vi "Autonomous Independent.vi"() -> ()   [LabVIEW 2023]
doc: "This VI is called when autonomous begins, and will automatically be terminated when autonomous ends. You can carry out timed or sensor driven robot movement independently without needing to return to the caller."
uses:
  <vilib>/Rock Robotics/WPI/ThirdParty/REV Robotics/REVLib/Typedef/Spark MAX Idle Mode.ctl
  <vilib>/Rock Robotics/WPI/SafetyOutput/WPI_SafetyOutputConfigMenu.ctl
  <vilib>/Rock Robotics/Network Tables/NT Read String.vi
  <vilib>/Rock Robotics/WPI/Utilities/WPI_GetSetVariantRefNum.vi
panel:
  out "Sensor Position 24":dbl
  out "Sensor Position 23":dbl
  out "Sensor Position 22":dbl
  out "Sensor Position 21":dbl
  out "Sensor Position 20":dbl
  out "Sensor Position 19":dbl
  out "Sensor Position 18":dbl
  out "Sensor Position 17":dbl
  out "Sensor Position 16":dbl
  out "Sensor Position 15":dbl
  out "Sensor Position 14":dbl
  out "Sensor Position 13":dbl
  out "Sensor Position 12":dbl
  out "Sensor Position 11":dbl
  out "Sensor Position 10":dbl
  out "Sensor Position 9":dbl
  out "Sensor Position 8":dbl
  out "Sensor Position 7":dbl
  out "?":dbl
  out "Sensor Position 6":dbl
  out "Sensor Position 5":dbl
  out "Sensor Position 4":dbl
  out "Sensor Position 3":dbl
  out "Sensor Position 2":dbl
  out "Sensor Position":dbl
  out "?":dbl
  # "Autonomous Independent.viBe sure to right-click and choose Data Operations>>Make Current Value default if you want to save the array values with the VI"
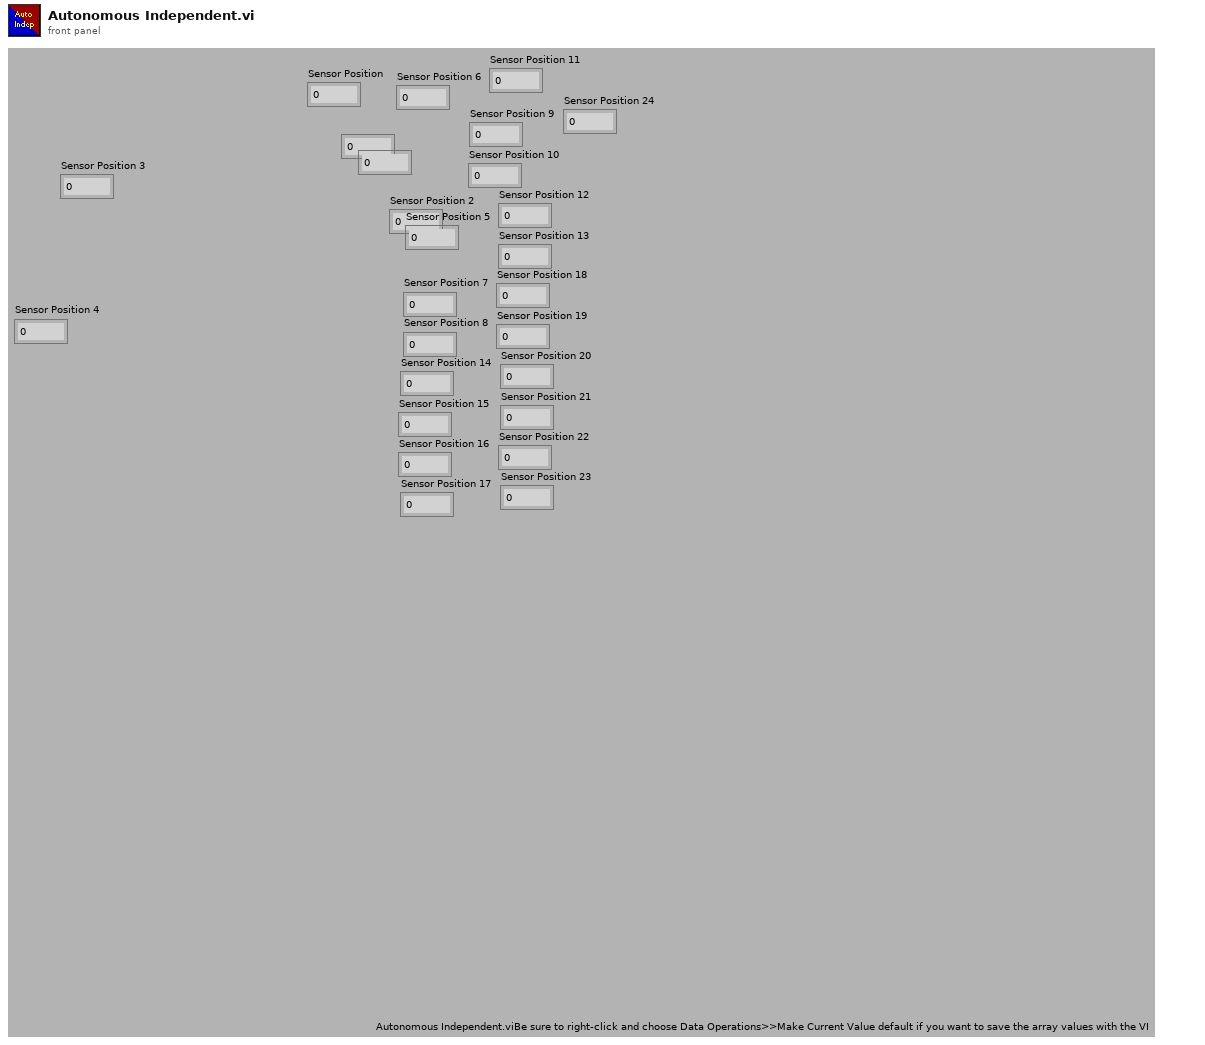
[diagram p1: front panel]
types:
  T1 = typedef "WPI_SafetyOutputConfigMenu.ctl" = enum16{"Enable", "Disable"}
  T2 = enum16{"ação 1", "ação 2", "ação 3", "ação 4", "ação 5", "ação 7", "ação 8"}
  T3 = typedef "Spark MAX Idle Mode.ctl" = enum16{"Coast", "Brake"}
  T4 = enum16{"ação 1", "ação 2", "ação 3", "ação 4", "ação 5"}
  T5 = typedef "WPI_RobotDriveDevRef.ctl" = cluster{"DevStatus":errorcluster, "Motors[]":T6[], "Square Inputs":bool, "Max Output":dbl}
  T6 = typedef "WPI_MotorControlDeviceRef.ctl" = cluster{"DeviceStatus":errorcluster, "Type":T7, "PWM":cluster{"PWM Channel":T8, "DeadBand":T9}, "CAN":cluster{"Device Number":u8, "SetOutput VI Ref":variant, "GetOutput VI Ref":variant, "Enable VI Ref":variant, "Disable VI Ref":variant, "Data":variant}, "Invert":bool, "DIO PWM":cluster{"PWM \"Enable\" Channel":T8, "DIOChannel":T10, "PWM Rate":dbl}}
  T7 = typedef "WPI_MotorControlType.ctl" = enum16{"PWM", "CAN", "DIO PWM"}
  T8 = typedef "FPGA_DIOPWMChannel.ctl" = enum8{"PWM 0", "PWM 1", "PWM 2", "PWM 3", "PWM 4", "PWM 5", "PWM 6", "PWM 7", "PWM 8", "PWM 9", "PWM MXP 0", "PWM MXP 1", "PWM MXP 2", "PWM MXP 3", "PWM MXP 4", "PWM MXP 5", "PWM MXP 6", "PWM MXP 7", "PWM MXP 8", "PWM MXP 9", "Invalid"}
  T9 = typedef "WPI_PWMDeadband.ctl" = cluster{"Name":string, "maxPositivePwm":i32, "minPositivePwm":i32, "centerPwm":i32, "maxNegativePwm":i32, "minNegativePwm":i32, "angularRange":u16}
  T10 = typedef "FPGA_DIOChannel.ctl" = enum8{"DIO 0", "DIO 1", "DIO 2", "DIO 3", "DIO 4", "DIO 5", "DIO 6", "DIO 7", "DIO 8", "DIO 9", "DIO MXP 0", "DIO MXP 1", "DIO MXP 2", "DIO MXP 3", "DIO MXP 4", "DIO MXP 5", "DIO MXP 6", "DIO MXP 7", "DIO MXP 8", "DIO MXP 9", "DIO MXP 10", "DIO MXP 11", "DIO MXP 12", "DIO MXP 13", "DIO MXP 14", "DIO MXP 15", "SPI Port CS1", "SPI Port CS2", "SPI Port CS3", "SPI Port MISO", "SPI Port MOSI", "Invalid"}
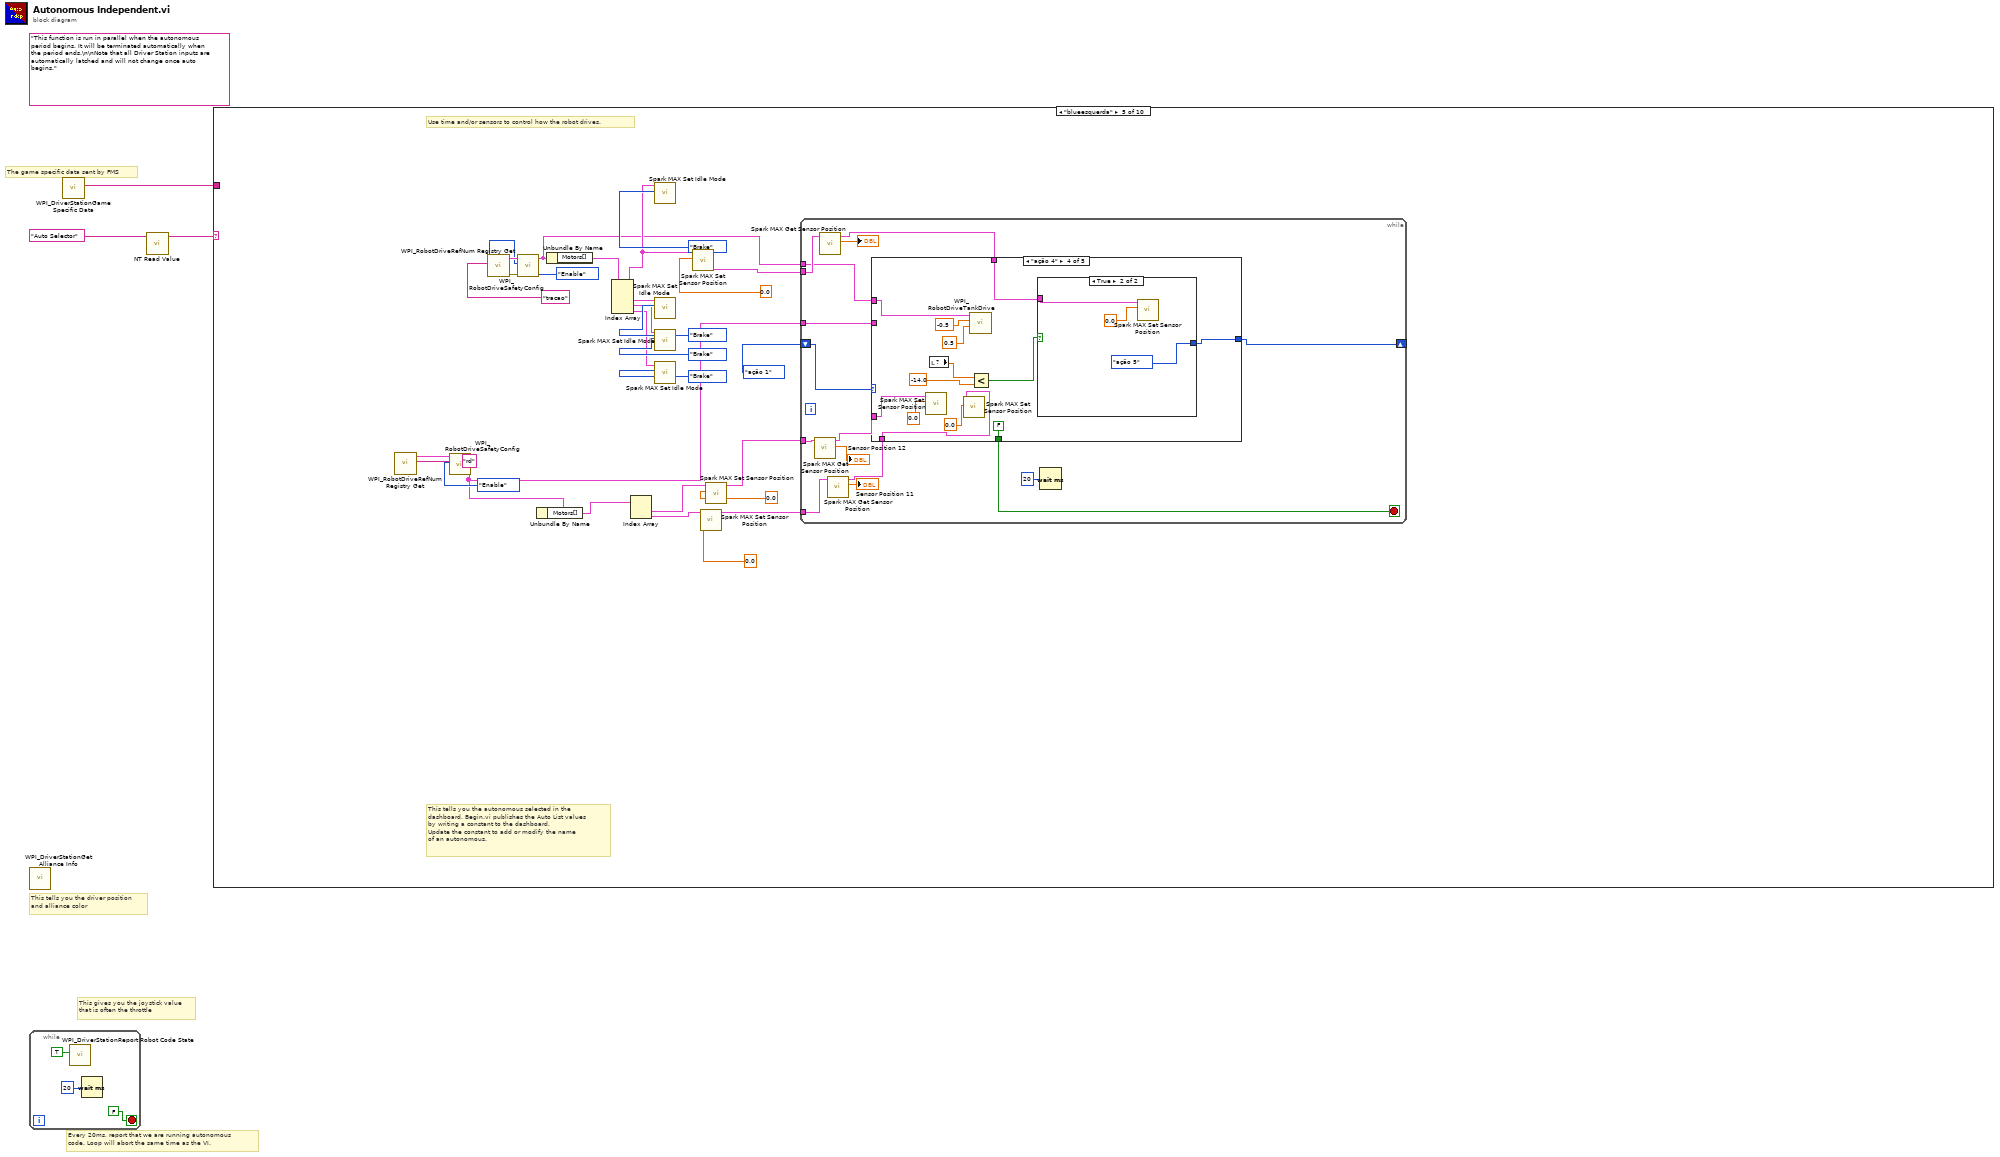
[diagram p0: block diagram]
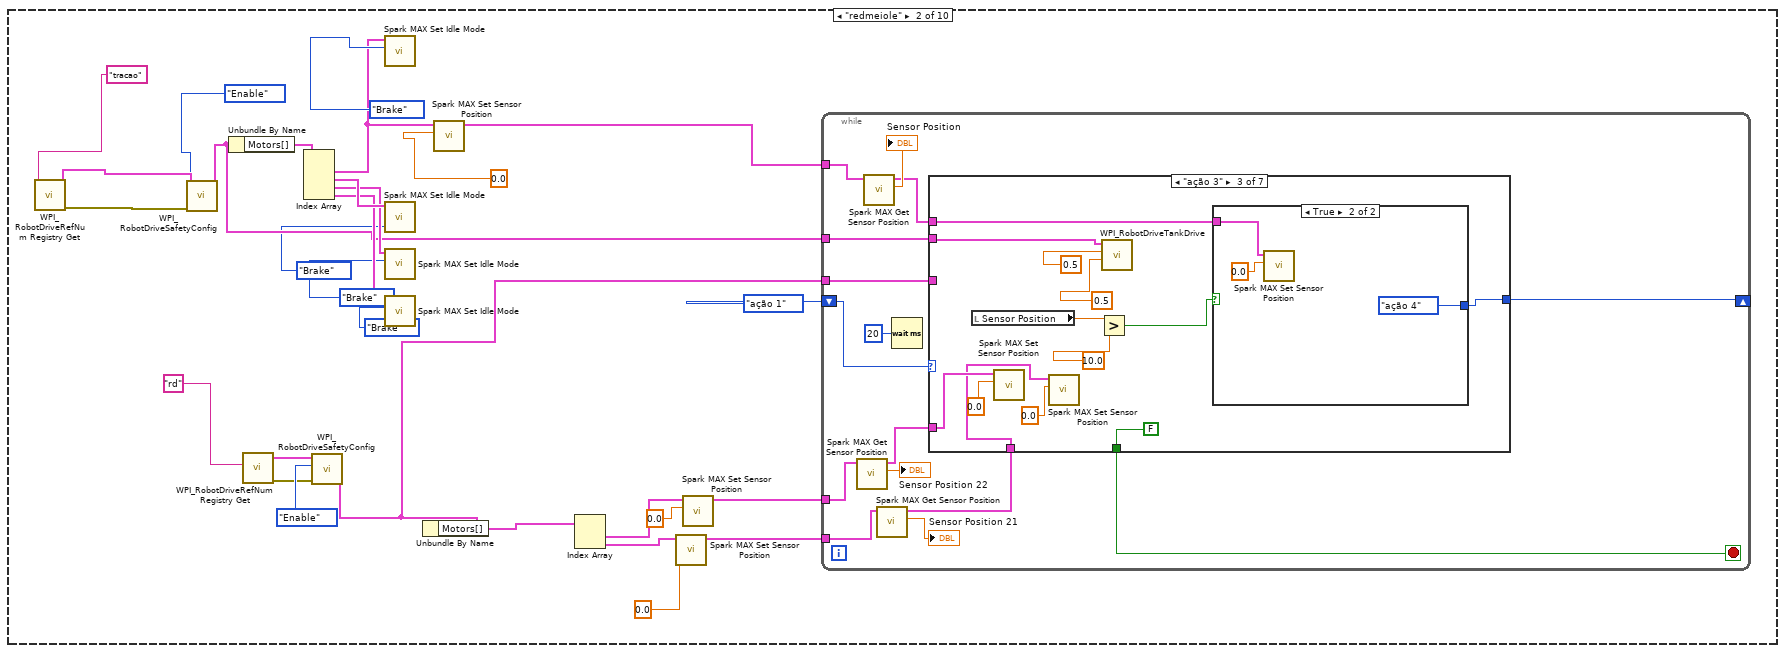
[diagram p3: hidden frame]
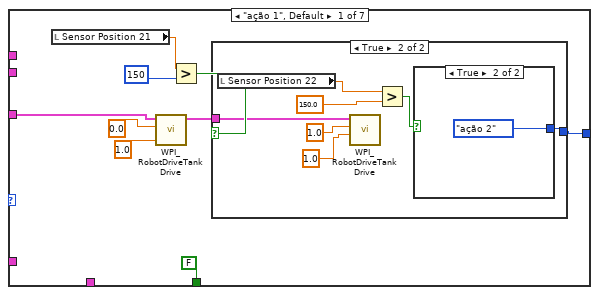
[diagram p4: hidden frame]
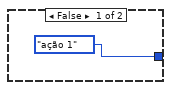
[diagram p5: hidden frame]
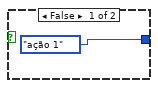
[diagram p6: hidden frame]
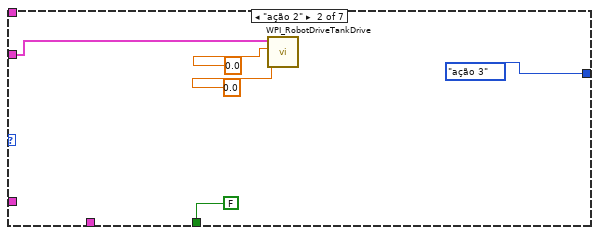
[diagram p7: hidden frame]
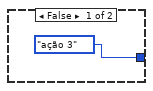
[diagram p8: hidden frame]
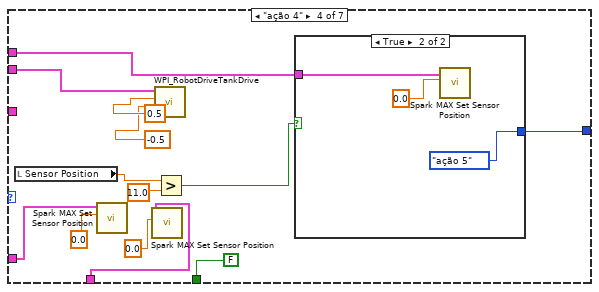
[diagram p9: hidden frame]
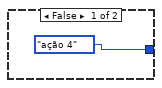
[diagram p10: hidden frame]
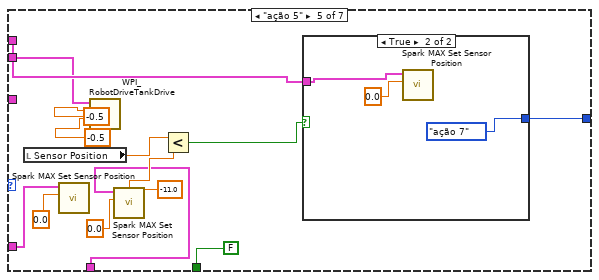
[diagram p11: hidden frame]
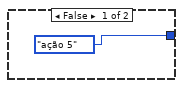
[diagram p12: hidden frame]
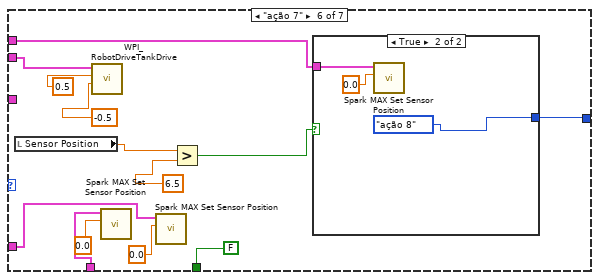
[diagram p13: hidden frame]
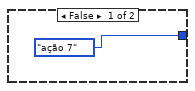
[diagram p14: hidden frame]
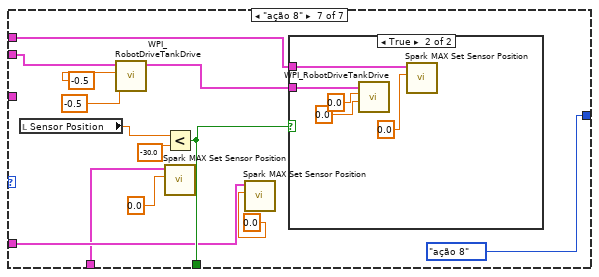
[diagram p15: hidden frame]
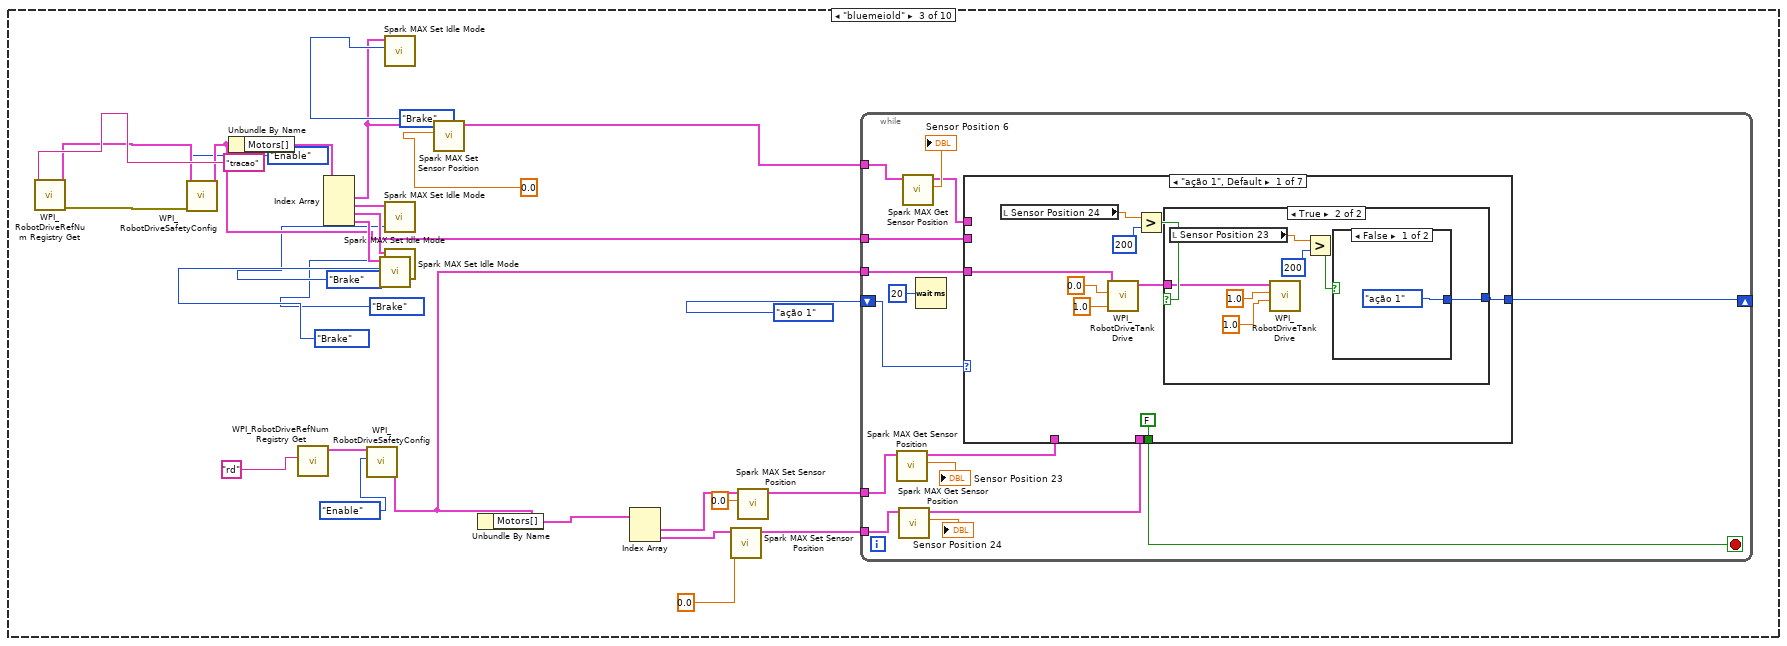
[diagram p17: hidden frame]
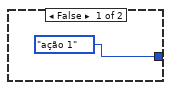
[diagram p18: hidden frame]
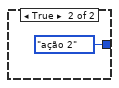
[diagram p19: hidden frame]
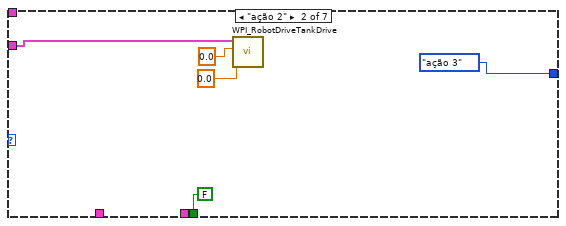
[diagram p20: hidden frame]
diagram:
  (unwired) "This function is run in parallel when the autonomous period begins. It will be terminated automatically when the period ends.\n\nNote that all Driver Station inputs are automatically latched and will not change once auto begins."
  # "The game specific data sent by FMS"
  # "This tells you the autonomous selected in the \ndashboard. Begin.vi publishes the Auto List values\nby writing a constant to the dashboard.\nUpdate the constant to add or modify the name\nof an autonomous."
  # "Every 20ms, report that we are running autonomous\ncode. Loop will abort the same time as the VI."
  # "This gives you the joystick value\nthat is often the throttle"
  # "Use time and/or sensors to control how the robot drives."
  # "This tells you the driver position\nand alliance color"
  n1 = call <vilib>:"WPI_DriverStationGet Alliance Info.vi"() -> ()  [unwired: 12 out]
  n2 = while {
    stop <- FALSE stop-if-true
    n3 = call <vilib>:"WPI_DriverStationReport Robot Code State.vi"("Autonomous"=TRUE) -> ()  [unwired: 10 in, 1 out]
    n4 = Wait (ms)(milliseconds to wait=u32 20) -> ()  [unwired: 1 out]
  }
  n5 = call <vilib>:"WPI_DriverStationGame Specific Data.vi"() -> ("Game Specific Data"=w1:string)  [unwired: 11 in]
  n6 = call-poly <vilib>:"NT Read Value.vi"("name"="Auto Selector" ("Name")) -> ("value"=w2:string)  [unwired: 8 in, 2 out]
  n7 = case shown="\"blueesquerda\"" w2 {
    tunnel: w1 -> [_ _ _ _ _ _ _ _ _ _]
    frame Default {
    }
    frame "redmeiole" {
      n8 = call <vilib>:"WPI_RobotDriveRefNum Registry Get.vi"("refnum name"="tracao") -> ("error out"=w34:errorcluster, "RobotDriveDevRef"=w33:T5)  [unwired: 9 in]
      n9 = call <vilib>:"WPI_RobotDriveSafetyConfig.vi"("error in (no error)"=w34, "mode"=WPI_SafetyOutputConfigMenu."Enable", "RobotDriveDevRef"=w33) -> ("RobotDriveDevRef"=w24:T5)  [unwired: 7 in, 1 out]
      n10 = Unbundle By Name(w24) -> ("Motors[]"=w32:T6[])
      n11 = call <vilib>:"WPI_RobotDriveRefNum Registry Get.vi"("refnum name"="rd") -> ("error out"=w7:errorcluster, "RobotDriveDevRef"=w13:T5)  [unwired: 9 in]
      n12 = Index Array(array=w32) -> (element #1=w25:T6, element #2=w29:T6, element #3=w28:T6, element #4=w27:T6)  [unwired: 4 in]
      n13 = call <vilib>:"WPI_RobotDriveSafetyConfig.vi"("error in (no error)"=w7, "mode"=WPI_SafetyOutputConfigMenu."Enable", "RobotDriveDevRef"=w13) -> ("RobotDriveDevRef"=w8:T5)  [unwired: 7 in, 1 out]
      n14 = call <vilib>:"Spark MAX Set Idle Mode.vi"("Idle Mode"=Spark_MAX_Idle_Mode."Brake", "MotorControlDeviceRef in"=w25) -> ()  [unwired: 8 in, 2 out]
      n15 = call <vilib>:"Spark MAX Set Idle Mode.vi"("Idle Mode"=Spark_MAX_Idle_Mode."Brake", "MotorControlDeviceRef in"=w29) -> ()  [unwired: 8 in, 2 out]
      n16 = call <vilib>:"Spark MAX Set Idle Mode.vi"("Idle Mode"=Spark_MAX_Idle_Mode."Brake", "MotorControlDeviceRef in"=w28) -> ()  [unwired: 8 in, 2 out]
      n17 = call <vilib>:"Spark MAX Set Idle Mode.vi"("Idle Mode"=Spark_MAX_Idle_Mode."Brake", "MotorControlDeviceRef in"=w27) -> ()  [unwired: 8 in, 2 out]
      n18 = Unbundle By Name(w8) -> ("Motors[]"=w18:T6[])
      n19 = call <vilib>:"Spark MAX Set Sensor Position.vi"("Position"=0.0, "MotorControlDeviceRef"=w25) -> ("MotorControlDeviceRef"=w23:T6)  [unwired: 8 in, 1 out]
      n20 = Index Array(array=w18) -> (element #1=w15:T6, element #2=w16:T6)  [unwired: 2 in]
      n21 = call <vilib>:"Spark MAX Set Sensor Position.vi"("Position"=0.0, "MotorControlDeviceRef"=w16) -> ("MotorControlDeviceRef"=w9:T6)  [unwired: 8 in, 1 out]
      n22 = call <vilib>:"Spark MAX Set Sensor Position.vi"("Position"=0.0, "MotorControlDeviceRef"=w15) -> ("MotorControlDeviceRef"=w10:T6)  [unwired: 8 in, 1 out]
      n23 = while {
        shift-right: [w48] -> _
        shift-left: T2."ação 1" -> [w49]
        tunnel: w24 -> [w47]
        tunnel: w23 -> [w45]
        tunnel: w10 -> [w42]
        tunnel: w9 -> [w41]
        tunnel: w8 -> [w38]
        stop <- w43 stop-if-true
        n24 = call <vilib>:"Spark MAX Get Sensor Position.vi"("MotorControlDevRef in"=w42) -> ("Sensor Position"=→"Sensor Position 22":dbl, "MotorControlDevRef out"=w37:T6)  [unwired: 7 in, 2 out]
        n25 = call <vilib>:"Spark MAX Get Sensor Position.vi"("MotorControlDevRef in"=w45) -> ("Sensor Position"=→"Sensor Position":dbl, "MotorControlDevRef out"=w44:T6)  [unwired: 7 in, 2 out]
        n26 = call <vilib>:"Spark MAX Get Sensor Position.vi"("MotorControlDevRef in"=w41) -> ("Sensor Position"=→"Sensor Position 21":dbl, "MotorControlDevRef out"=w36:T6)  [unwired: 7 in, 2 out]
        n27 = Wait (ms)(milliseconds to wait=u32 20) -> ()  [unwired: 1 out]
        n28 = case shown="\"ação 3\"" w49 {
          tunnel: [w54 T2."ação 3" w80 w97 w114 w131 T2."ação 8"] -> w48
          tunnel: w47 -> [_ _ w87 w104 w118 w138 w155]
          tunnel: w44 -> [_ _ w81 w98 w121 w132 w143]
          tunnel: [FALSE FALSE FALSE FALSE FALSE FALSE w149] -> w43
          tunnel: w38 -> [w51 w70 _ _ _ _ _]
          tunnel: w37 -> [_ _ w76 w92 w110 w126 w147]
          tunnel: w36 -> [_ _ w75 w93 w109 w127 w144]
          frame "ação 1", Default {
            n29 = local read "Sensor Position 21"() -> (w52:dbl)
            n30 = call <vilib>:"WPI_RobotDriveTankDrive.vi"("Right axis value"=1.0, "Left axis value"=0.0, "RobotDriveDevRef"=w51) -> ("RobotDriveDevRef"=w57:T5)  [unwired: 6 in, 2 out]
            n31 = Greater?(x=w52, y=u32 150) -> (0:w55:bool)
            n32 = case shown="True" w55 {
              tunnel: w57 -> [_ w65]
              tunnel: [T2."ação 1" w62] -> w54
              frame False {
              }
              frame True {
                n33 = local read "Sensor Position 22"() -> (w64:dbl)
                n34 = call <vilib>:"WPI_RobotDriveTankDrive.vi"("Right axis value"=1.0 ("Left axis value"), "Left axis value"=1.0 ("Right axis value"), "RobotDriveDevRef"=w65) -> ()  [unwired: 6 in, 3 out]
                n35 = Greater?(x=w64, y=150.0) -> (0:w63:bool)
                n36 = case shown="True" w63 {
                  tunnel: [T2."ação 1" T2."ação 2"] -> w62
                  frame False {
                  }
                  frame True {
                  }
                }
              }
            }
          }
          frame "ação 2" {
            n37 = call <vilib>:"WPI_RobotDriveTankDrive.vi"("Right axis value"=0.0, "Left axis value"=0.0, "RobotDriveDevRef"=w70) -> ()  [unwired: 6 in, 3 out]
          }
          frame "ação 3" {
            n38 = local read "Sensor Position"() -> (w83:dbl)
            n39 = call <vilib>:"Spark MAX Set Sensor Position.vi"("Position"=0.0, "MotorControlDeviceRef"=w76) -> ()  [unwired: 8 in, 2 out]
            n40 = call <vilib>:"Spark MAX Set Sensor Position.vi"("Position"=0.0, "MotorControlDeviceRef"=w75) -> ()  [unwired: 8 in, 2 out]
            n41 = Greater?(x=w83, y=10.0) -> (0:w84:bool)
            n42 = call <vilib>:"WPI_RobotDriveTankDrive.vi"("Right axis value"=0.5 ("Left axis value"), "Left axis value"=0.5, "RobotDriveDevRef"=w87) -> ()  [unwired: 6 in, 3 out]
            n43 = case shown="True" w84 {
              tunnel: w81 -> [_ w91]
              tunnel: [T2."ação 3" T2."ação 4"] -> w80
              frame False {
              }
              frame True {
                n44 = call <vilib>:"Spark MAX Set Sensor Position.vi"("Position"=0.0, "MotorControlDeviceRef"=w91) -> ()  [unwired: 8 in, 2 out]
              }
            }
          }
          frame "ação 4" {
            n45 = local read "Sensor Position"() -> (w101:dbl)
            n46 = call <vilib>:"Spark MAX Set Sensor Position.vi"("Position"=0.0, "MotorControlDeviceRef"=w92) -> ()  [unwired: 8 in, 2 out]
            n47 = call <vilib>:"Spark MAX Set Sensor Position.vi"("Position"=0.0, "MotorControlDeviceRef"=w93) -> ()  [unwired: 8 in, 2 out]
            n48 = call <vilib>:"WPI_RobotDriveTankDrive.vi"("Right axis value"=-0.5 ("Left axis value"), "Left axis value"=0.5, "RobotDriveDevRef"=w104) -> ()  [unwired: 6 in, 3 out]
            n49 = Greater?(x=w101, y=11.0) -> (0:w99:bool)
            n50 = case shown="True" w99 {
              tunnel: w98 -> [_ w108]
              tunnel: [T2."ação 4" T2."ação 5"] -> w97
              frame False {
              }
              frame True {
                n51 = call <vilib>:"Spark MAX Set Sensor Position.vi"("Position"=0.0, "MotorControlDeviceRef"=w108) -> ()  [unwired: 8 in, 2 out]
              }
            }
          }
          frame "ação 5" {
            n52 = local read "Sensor Position"() -> (w117:dbl)
            n53 = call <vilib>:"Spark MAX Set Sensor Position.vi"("Position"=0.0, "MotorControlDeviceRef"=w110) -> ()  [unwired: 8 in, 2 out]
            n54 = call <vilib>:"WPI_RobotDriveTankDrive.vi"("Right axis value"=-0.5 ("Left axis value"), "Left axis value"=-0.5, "RobotDriveDevRef"=w118) -> ()  [unwired: 6 in, 3 out]
            n55 = call <vilib>:"Spark MAX Set Sensor Position.vi"("Position"=0.0, "MotorControlDeviceRef"=w109) -> ()  [unwired: 8 in, 2 out]
            n56 = Less?(x=w117, y=-11.0) -> (x < y?=w115:bool)
            n57 = case shown="True" w115 {
              tunnel: w121 -> [_ w124]
              tunnel: [T2."ação 5" T2."ação 7"] -> w114
              frame False {
              }
              frame True {
                n58 = call <vilib>:"Spark MAX Set Sensor Position.vi"("Position"=0.0, "MotorControlDeviceRef"=w124) -> ()  [unwired: 8 in, 2 out]
              }
            }
          }
          frame "ação 7" {
            n59 = local read "Sensor Position"() -> (w135:dbl)
            n60 = call <vilib>:"WPI_RobotDriveTankDrive.vi"("Right axis value"=-0.5 ("Left axis value"), "Left axis value"=0.5, "RobotDriveDevRef"=w138) -> ()  [unwired: 6 in, 3 out]
            n61 = call <vilib>:"Spark MAX Set Sensor Position.vi"("Position"=0.0, "MotorControlDeviceRef"=w127) -> ()  [unwired: 8 in, 2 out]
            n62 = call <vilib>:"Spark MAX Set Sensor Position.vi"("Position"=0.0, "MotorControlDeviceRef"=w126) -> ()  [unwired: 8 in, 2 out]
            n63 = Greater?(x=w135, y=6.5) -> (0:w133:bool)
            n64 = case shown="True" w133 {
              tunnel: w132 -> [_ w142]
              tunnel: [T2."ação 7" T2."ação 8"] -> w131
              frame False {
              }
              frame True {
                n65 = call <vilib>:"Spark MAX Set Sensor Position.vi"("Position"=0.0, "MotorControlDeviceRef"=w142) -> ()  [unwired: 8 in, 2 out]
              }
            }
          }
          frame "ação 8" {
            n66 = local read "Sensor Position"() -> (w152:dbl)
            n67 = call <vilib>:"WPI_RobotDriveTankDrive.vi"("Right axis value"=-0.5 ("Left axis value"), "Left axis value"=-0.5, "RobotDriveDevRef"=w155) -> ("RobotDriveDevRef"=w150:T5)  [unwired: 6 in, 2 out]
            n68 = Less?(x=w152, y=-30.0) -> (x < y?=w149:bool)
            n69 = call <vilib>:"Spark MAX Set Sensor Position.vi"("Position"=0.0, "MotorControlDeviceRef"=w144) -> ()  [unwired: 8 in, 2 out]
            n70 = call <vilib>:"Spark MAX Set Sensor Position.vi"("Position"=0.0, "MotorControlDeviceRef"=w147) -> ()  [unwired: 8 in, 2 out]
            n71 = case shown="True" w149 {
              tunnel: w150 -> [_ w160]
              tunnel: w143 -> [_ w157]
              frame False {
              }
              frame True {
                n72 = call <vilib>:"WPI_RobotDriveTankDrive.vi"("Right axis value"=0.0 ("Left axis value"), "Left axis value"=0.0, "RobotDriveDevRef"=w160) -> ()  [unwired: 6 in, 3 out]
                n73 = call <vilib>:"Spark MAX Set Sensor Position.vi"("Position"=0.0, "MotorControlDeviceRef"=w157) -> ()  [unwired: 8 in, 2 out]
              }
            }
          }
        }
      }
    }
    frame "bluemeiold" {
      n74 = call <vilib>:"WPI_RobotDriveRefNum Registry Get.vi"("refnum name"="tracao") -> ("error out"=w187:errorcluster, "RobotDriveDevRef"=w186:T5)  [unwired: 9 in]
      n75 = call <vilib>:"WPI_RobotDriveSafetyConfig.vi"("error in (no error)"=w187, "mode"=WPI_SafetyOutputConfigMenu."Enable", "RobotDriveDevRef"=w186) -> ("RobotDriveDevRef"=w177:T5)  [unwired: 7 in, 1 out]
      n76 = Unbundle By Name(w177) -> ("Motors[]"=w185:T6[])
      n77 = call <vilib>:"WPI_RobotDriveRefNum Registry Get.vi"("refnum name"="rd") -> ("RobotDriveDevRef"=w165:T5)  [unwired: 9 in, 1 out]
      n78 = Index Array(array=w185) -> (element #1=w178:T6, element #2=w182:T6, element #3=w181:T6, element #4=w180:T6)  [unwired: 4 in]
      n79 = call <vilib>:"WPI_RobotDriveSafetyConfig.vi"("mode"=WPI_SafetyOutputConfigMenu."Enable", "RobotDriveDevRef"=w165) -> ("RobotDriveDevRef"=w161:T5)  [unwired: 8 in, 1 out]
      n80 = call <vilib>:"Spark MAX Set Idle Mode.vi"("Idle Mode"=Spark_MAX_Idle_Mode."Brake", "MotorControlDeviceRef in"=w180) -> ()  [unwired: 8 in, 2 out]
      n81 = call <vilib>:"Spark MAX Set Idle Mode.vi"("Idle Mode"=Spark_MAX_Idle_Mode."Brake", "MotorControlDeviceRef in"=w178) -> ()  [unwired: 8 in, 2 out]
      n82 = call <vilib>:"Spark MAX Set Idle Mode.vi"("Idle Mode"=Spark_MAX_Idle_Mode."Brake", "MotorControlDeviceRef in"=w182) -> ()  [unwired: 8 in, 2 out]
      n83 = call <vilib>:"Spark MAX Set Idle Mode.vi"("Idle Mode"=Spark_MAX_Idle_Mode."Brake", "MotorControlDeviceRef in"=w181) -> ()  [unwired: 8 in, 2 out]
      n84 = call <vilib>:"Spark MAX Set Sensor Position.vi"("Position"=0.0, "MotorControlDeviceRef"=w178) -> ("MotorControlDeviceRef"=w176:T6)  [unwired: 8 in, 1 out]
      n85 = Unbundle By Name(w161) -> ("Motors[]"=w171:T6[])
      n86 = Index Array(array=w171) -> (element #1=w168:T6, element #2=w169:T6)  [unwired: 2 in]
      n87 = call <vilib>:"Spark MAX Set Sensor Position.vi"("Position"=0.0, "MotorControlDeviceRef"=w169) -> ("MotorControlDeviceRef"=w162:T6)  [unwired: 8 in, 1 out]
      n88 = call <vilib>:"Spark MAX Set Sensor Position.vi"("Position"=0.0, "MotorControlDeviceRef"=w168) -> ("MotorControlDeviceRef"=w163:T6)  [unwired: 8 in, 1 out]
      n89 = while {
        shift-right: [w201] -> _
        shift-left: T2."ação 1" -> [w202]
        tunnel: w177 -> [w200]
        tunnel: w176 -> [w198]
        tunnel: w163 -> [w195]
        tunnel: w162 -> [w194]
        tunnel: w161 -> [w191]
        stop <- w196 stop-if-true
        n90 = call <vilib>:"Spark MAX Get Sensor Position.vi"("MotorControlDevRef in"=w195) -> ("Sensor Position"=→"Sensor Position 23":dbl, "MotorControlDevRef out"=w190:T6)  [unwired: 7 in, 2 out]
        n91 = call <vilib>:"Spark MAX Get Sensor Position.vi"("MotorControlDevRef in"=w194) -> ("Sensor Position"=→"Sensor Position 24":dbl, "MotorControlDevRef out"=w189:T6)  [unwired: 7 in, 2 out]
        n92 = call <vilib>:"Spark MAX Get Sensor Position.vi"("MotorControlDevRef in"=w198) -> ("Sensor Position"=→"Sensor Position 6":dbl, "MotorControlDevRef out"=w197:T6)  [unwired: 7 in, 2 out]
        n93 = Wait (ms)(milliseconds to wait=u32 20) -> ()  [unwired: 1 out]
        n94 = case shown="\"ação 1\", Default" w202 {
          tunnel: [w207 T2."ação 3" w233 w250 w267 w284 T2."ação 8"] -> w201
          tunnel: w200 -> [_ _ w240 w257 w271 w291 w308]
          tunnel: w197 -> [_ _ w234 w251 w274 w285 w296]
          tunnel: [FALSE FALSE FALSE FALSE FALSE FALSE w302] -> w196
          tunnel: w191 -> [w204 w223 _ _ _ _ _]
          tunnel: w190 -> [_ _ w229 w246 w265 w282 w298]
          tunnel: w189 -> [_ _ w228 w245 w264 w281 w297]
          frame "ação 1", Default {
            n95 = local read "Sensor Position 24"() -> (w205:dbl)
            n96 = call <vilib>:"WPI_RobotDriveTankDrive.vi"("Right axis value"=1.0, "Left axis value"=0.0, "RobotDriveDevRef"=w204) -> ("RobotDriveDevRef"=w210:T5)  [unwired: 6 in, 2 out]
            n97 = Greater?(x=w205, y=u32 200) -> (0:w208:bool)
            n98 = case shown="True" w208 {
              tunnel: w210 -> [_ w218]
              tunnel: [T2."ação 1" w214] -> w207
              frame False {
              }
              frame True {
                n99 = local read "Sensor Position 23"() -> (w217:dbl)
                n100 = call <vilib>:"WPI_RobotDriveTankDrive.vi"("Right axis value"=1.0 ("Left axis value"), "Left axis value"=1.0 ("Right axis value"), "RobotDriveDevRef"=w218) -> ()  [unwired: 6 in, 3 out]
                n101 = Greater?(x=w217, y=u32 200) -> (0:w215:bool)
                n102 = case shown="False" w215 {
                  tunnel: [T2."ação 1" T2."ação 2"] -> w214
                  frame False {
                  }
                  frame True {
                  }
                }
              }
            }
          }
          frame "ação 2" {
            n103 = call <vilib>:"WPI_RobotDriveTankDrive.vi"("Right axis value"=0.0, "Left axis value"=0.0, "RobotDriveDevRef"=w223) -> ()  [unwired: 6 in, 3 out]
          }
          frame "ação 3" {
            n104 = local read "Sensor Position 6"() -> (w236:dbl)
            n105 = call <vilib>:"Spark MAX Set Sensor Position.vi"("Position"=0.0, "MotorControlDeviceRef"=w229) -> ()  [unwired: 8 in, 2 out]
            n106 = Greater?(x=w236, y=10.0) -> (0:w237:bool)
            n107 = call <vilib>:"WPI_RobotDriveTankDrive.vi"("Right axis value"=0.5 ("Left axis value"), "Left axis value"=0.5, "RobotDriveDevRef"=w240) -> ()  [unwired: 6 in, 3 out]
            n108 = call <vilib>:"Spark MAX Set Sensor Position.vi"("Position"=0.0, "MotorControlDeviceRef"=w228) -> ()  [unwired: 8 in, 2 out]
            n109 = case shown="True" w237 {
              tunnel: w234 -> [_ w244]
              tunnel: [T2."ação 3" T2."ação 4"] -> w233
              frame False {
              }
              frame True {
                n110 = call <vilib>:"Spark MAX Set Sensor Position.vi"("Position"=0.0, "MotorControlDeviceRef"=w244) -> ()  [unwired: 8 in, 2 out]
              }
            }
          }
          frame "ação 4" {
            n111 = local read "Sensor Position 6"() -> (w254:dbl)
            n112 = call <vilib>:"WPI_RobotDriveTankDrive.vi"("Right axis value"=0.5 ("Left axis value"), "Left axis value"=-0.5, "RobotDriveDevRef"=w257) -> ()  [unwired: 6 in, 3 out]
            n113 = Less?(x=w254, y=-11.0) -> (x < y?=w252:bool)
            n114 = call <vilib>:"Spark MAX Set Sensor Position.vi"("Position"=0.0, "MotorControlDeviceRef"=w246) -> ()  [unwired: 8 in, 2 out]
            n115 = call <vilib>:"Spark MAX Set Sensor Position.vi"("Position"=0.0, "MotorControlDeviceRef"=w245) -> ()  [unwired: 8 in, 2 out]
            n116 = case shown="True" w252 {
              tunnel: w251 -> [_ w261]
              tunnel: [T2."ação 4" T2."ação 5"] -> w250
              frame False {
              }
              frame True {
                n117 = call <vilib>:"Spark MAX Set Sensor Position.vi"("Position"=0.0, "MotorControlDeviceRef"=w261) -> ()  [unwired: 8 in, 2 out]
              }
            }
          }
          frame "ação 5" {
            n118 = local read "Sensor Position 6"() -> (w270:dbl)
            n119 = call <vilib>:"WPI_RobotDriveTankDrive.vi"("Right axis value"=-0.5 ("Left axis value"), "Left axis value"=-0.5, "RobotDriveDevRef"=w271) -> ()  [unwired: 6 in, 3 out]
            n120 = Less?(x=w270, y=-11.0) -> (x < y?=w268:bool)
            n121 = call <vilib>:"Spark MAX Set Sensor Position.vi"("Position"=0.0, "MotorControlDeviceRef"=w265) -> ()  [unwired: 8 in, 2 out]
            n122 = call <vilib>:"Spark MAX Set Sensor Position.vi"("Position"=0.0, "MotorControlDeviceRef"=w264) -> ()  [unwired: 8 in, 2 out]
            n123 = case shown="True" w268 {
              tunnel: w274 -> [_ w277]
              tunnel: [T2."ação 5" T2."ação 7"] -> w267
              frame False {
              }
              frame True {
                n124 = call <vilib>:"Spark MAX Set Sensor Position.vi"("Position"=0.0, "MotorControlDeviceRef"=w277) -> ()  [unwired: 8 in, 2 out]
              }
            }
          }
          frame "ação 7" {
            n125 = local read "Sensor Position 6"() -> (w288:dbl)
            n126 = call <vilib>:"WPI_RobotDriveTankDrive.vi"("Right axis value"=0.5 ("Left axis value"), "Left axis value"=-0.5, "RobotDriveDevRef"=w291) -> ()  [unwired: 6 in, 3 out]
            n127 = Less?(x=w288, y=-6.5) -> (x < y?=w286:bool)
            n128 = call <vilib>:"Spark MAX Set Sensor Position.vi"("Position"=0.0, "MotorControlDeviceRef"=w282) -> ()  [unwired: 8 in, 2 out]
            n129 = call <vilib>:"Spark MAX Set Sensor Position.vi"("Position"=0.0, "MotorControlDeviceRef"=w281) -> ()  [unwired: 8 in, 2 out]
            n130 = case shown="True" w286 {
              tunnel: w285 -> [_ w295]
              tunnel: [T2."ação 7" T2."ação 8"] -> w284
              frame False {
              }
              frame True {
                n131 = call <vilib>:"Spark MAX Set Sensor Position.vi"("Position"=0.0, "MotorControlDeviceRef"=w295) -> ()  [unwired: 8 in, 2 out]
              }
            }
          }
          frame "ação 8" {
            n132 = local read "Sensor Position 6"() -> (w305:dbl)
            n133 = call <vilib>:"Spark MAX Set Sensor Position.vi"("Position"=0.0, "MotorControlDeviceRef"=w298) -> ()  [unwired: 8 in, 2 out]
            n134 = call <vilib>:"WPI_RobotDriveTankDrive.vi"("Right axis value"=-0.5 ("Left axis value"), "Left axis value"=-0.5, "RobotDriveDevRef"=w308) -> ("RobotDriveDevRef"=w303:T5)  [unwired: 6 in, 2 out]
            n135 = Less?(x=w305, y=-30.0) -> (x < y?=w302:bool)
            n136 = call <vilib>:"Spark MAX Set Sensor Position.vi"("Position"=0.0, "MotorControlDeviceRef"=w297) -> ()  [unwired: 8 in, 2 out]
            n137 = case shown="True" w302 {
              tunnel: w303 -> [_ w313]
              tunnel: w296 -> [_ w310]
              frame False {
              }
              frame True {
                n138 = call <vilib>:"WPI_RobotDriveTankDrive.vi"("Right axis value"=0.0 ("Left axis value"), "Left axis value"=0.0, "RobotDriveDevRef"=w313) -> ()  [unwired: 6 in, 3 out]
                n139 = call <vilib>:"Spark MAX Set Sensor Position.vi"("Position"=0.0, "MotorControlDeviceRef"=w310) -> ()  [unwired: 8 in, 2 out]
              }
            }
          }
        }
      }
    }
    frame "reddireita" {
      n140 = call <vilib>:"WPI_RobotDriveRefNum Registry Get.vi"("refnum name"="rd") -> ("RobotDriveDevRef"=w323:T5)  [unwired: 9 in, 1 out]
      n141 = call <vilib>:"WPI_RobotDriveSafetyConfig.vi"("mode"=WPI_SafetyOutputConfigMenu."Enable", "RobotDriveDevRef"=w323) -> ("RobotDriveDevRef"=w314:T5)  [unwired: 8 in, 1 out]
      n142 = call <vilib>:"WPI_RobotDriveRefNum Registry Get.vi"("refnum name"="tracao") -> ("error out"=w340:errorcluster, "RobotDriveDevRef"=w339:T5)  [unwired: 9 in]
      n143 = call <vilib>:"WPI_RobotDriveSafetyConfig.vi"("error in (no error)"=w340, "mode"=WPI_SafetyOutputConfigMenu."Enable", "RobotDriveDevRef"=w339) -> ("RobotDriveDevRef"=w325:T5)  [unwired: 7 in, 1 out]
      n144 = Unbundle By Name(w314) -> ("Motors[]"=w321:T6[])
      n145 = Unbundle By Name(w325) -> ("Motors[]"=w337:T6[])
      n146 = Index Array(array=w337) -> (element #1=w329:T6, element #2=w332:T6, element #3=w331:T6, element #4=w330:T6)  [unwired: 4 in]
      n147 = Index Array(array=w321) -> (element #1=w317:T6, element #2=w318:T6)  [unwired: 2 in]
      n148 = call <vilib>:"Spark MAX Set Idle Mode.vi"("Idle Mode"=Spark_MAX_Idle_Mode."Brake", "MotorControlDeviceRef in"=w329) -> ()  [unwired: 8 in, 2 out]
      n149 = call <vilib>:"Spark MAX Set Idle Mode.vi"("Idle Mode"=Spark_MAX_Idle_Mode."Brake", "MotorControlDeviceRef in"=w332) -> ()  [unwired: 8 in, 2 out]
      n150 = call <vilib>:"Spark MAX Set Idle Mode.vi"("Idle Mode"=Spark_MAX_Idle_Mode."Brake", "MotorControlDeviceRef in"=w331) -> ()  [unwired: 8 in, 2 out]
      n151 = call <vilib>:"Spark MAX Set Idle Mode.vi"("Idle Mode"=Spark_MAX_Idle_Mode."Brake", "MotorControlDeviceRef in"=w330) -> ()  [unwired: 8 in, 2 out]
      n152 = call <vilib>:"Spark MAX Set Sensor Position.vi"("Position"=0.0, "MotorControlDeviceRef"=w329) -> ("MotorControlDeviceRef"=w327:T6)  [unwired: 8 in, 1 out]
      n153 = call <vilib>:"Spark MAX Set Sensor Position.vi"("Position"=0.0, "MotorControlDeviceRef"=w318) -> ("MotorControlDeviceRef"=w319:T6)  [unwired: 8 in, 1 out]
      n154 = call <vilib>:"Spark MAX Set Sensor Position.vi"("Position"=0.0, "MotorControlDeviceRef"=w317) -> ("MotorControlDeviceRef"=w315:T6)  [unwired: 8 in, 1 out]
      n155 = while {
        shift-right: [w350] -> _
        shift-left: T4."ação 1" -> [w355]
        tunnel: w327 -> [w353]
        tunnel: w325 -> [w351]
        tunnel: w319 -> [w348]
        tunnel: w315 -> [w346]
        tunnel: w314 -> [w344]
        stop <- w354 stop-if-true
        n156 = call <vilib>:"Spark MAX Get Sensor Position.vi"("MotorControlDevRef in"=w353) -> ("Sensor Position"=→"?":dbl, "MotorControlDevRef out"=w349:T6)  [unwired: 7 in, 2 out]
        n157 = call <vilib>:"Spark MAX Get Sensor Position.vi"("MotorControlDevRef in"=w346) -> ("Sensor Position"=→"Sensor Position 10":dbl, "MotorControlDevRef out"=w343:T6)  [unwired: 7 in, 2 out]
        n158 = call <vilib>:"Spark MAX Get Sensor Position.vi"("MotorControlDevRef in"=w348) -> ("Sensor Position"=→"Sensor Position 9":dbl, "MotorControlDevRef out"=w342:T6)  [unwired: 7 in, 2 out]
        n159 = case shown="\"ação 4\"" w355 {
          tunnel: [FALSE FALSE FALSE FALSE w425] -> w354
          tunnel: [w361 T4."ação 3" w389 w406 T4."ação 5"] -> w350
          tunnel: w351 -> [_ _ w391 w408 w422]
          tunnel: w349 -> [w357 _ w388 w405 w418]
          tunnel: w344 -> [w358 w379 _ _ _]
          tunnel: w343 -> [_ _ w385 w402 w419]
          tunnel: w342 -> [_ _ w384 w401 _]
          frame "ação 1", Default {
            n160 = local read "Sensor Position 9"() -> (w360:dbl)
            n161 = call <vilib>:"WPI_RobotDriveTankDrive.vi"("Right axis value"=1.0, "Left axis value"=0.0, "RobotDriveDevRef"=w358) -> ("RobotDriveDevRef"=w364:T5)  [unwired: 6 in, 2 out]
            n162 = Greater?(x=w360, y=150.0) -> (0:w363:bool)
            n163 = case shown="True" w363 {
              tunnel: w364 -> [_ w374]
              tunnel: [T4."ação 1" w370] -> w361
              tunnel: w357 -> [_ w369]
              frame False {
              }
              frame True {
                n164 = local read "Sensor Position 10"() -> (w373:dbl)
                n165 = call <vilib>:"Spark MAX Set Sensor Position.vi"("Position"=0.0, "MotorControlDeviceRef"=w369) -> ()  [unwired: 8 in, 2 out]
                n166 = call <vilib>:"WPI_RobotDriveTankDrive.vi"("Right axis value"=1.0 ("Left axis value"), "Left axis value"=1.0 ("Right axis value"), "RobotDriveDevRef"=w374) -> ()  [unwired: 6 in, 3 out]
                n167 = Greater?(x=w373, y=150.0) -> (0:w371:bool)
                n168 = case shown="True" w371 {
                  tunnel: [T4."ação 1" T4."ação 2"] -> w370
                  frame False {
                  }
                  frame True {
                  }
                }
              }
            }
          }
          frame "ação 2" {
            n169 = call <vilib>:"WPI_RobotDriveTankDrive.vi"("Right axis value"=0.0 ("Left axis value"), "Left axis value"=0.0, "RobotDriveDevRef"=w379) -> ()  [unwired: 6 in, 3 out]
          }
          frame "ação 3" {
            n170 = call <vilib>:"Spark MAX Set Sensor Position.vi"("Position"=0.0, "MotorControlDeviceRef"=w385) -> ()  [unwired: 8 in, 2 out]
            n171 = local read item#?() -> (w390:dbl)
            n172 = call <vilib>:"Spark MAX Set Sensor Position.vi"("Position"=0.0, "MotorControlDeviceRef"=w384) -> ()  [unwired: 8 in, 2 out]
            n173 = Greater?(x=w390, y=14.0) -> (0:w394:bool)
            n174 = call <vilib>:"WPI_RobotDriveTankDrive.vi"("Right axis value"=0.5 ("Left axis value"), "Left axis value"=0.5, "RobotDriveDevRef"=w391) -> ()  [unwired: 6 in, 3 out]
            n175 = case shown="True" w394 {
              tunnel: [T4."ação 3" T4."ação 4"] -> w389
              tunnel: w388 -> [_ w398]
              frame False {
              }
              frame True {
                n176 = call <vilib>:"Spark MAX Set Sensor Position.vi"("Position"=0.0, "MotorControlDeviceRef"=w398) -> ()  [unwired: 8 in, 2 out]
              }
            }
          }
          frame "ação 4" {
            n177 = call <vilib>:"Spark MAX Set Sensor Position.vi"("Position"=0.0, "MotorControlDeviceRef"=w402) -> ()  [unwired: 8 in, 2 out]
            n178 = local read item#?() -> (w407:dbl)
            n179 = call <vilib>:"Spark MAX Set Sensor Position.vi"("Position"=0.0, "MotorControlDeviceRef"=w401) -> ()  [unwired: 8 in, 2 out]
            n180 = call <vilib>:"WPI_RobotDriveTankDrive.vi"("Right axis value"=-0.5 ("Left axis value"), "Left axis value"=0.5, "RobotDriveDevRef"=w408) -> ()  [unwired: 6 in, 3 out]
            n181 = Greater?(x=w407, y=14.0) -> (0:w410:bool)
            n182 = case shown="True" w410 {
              tunnel: [T4."ação 4" T4."ação 5"] -> w406
              tunnel: w405 -> [_ w415]
              frame False {
              }
              frame True {
                n183 = call <vilib>:"Spark MAX Set Sensor Position.vi"("Position"=0.0, "MotorControlDeviceRef"=w415) -> ()  [unwired: 8 in, 2 out]
              }
            }
          }
          frame "ação 5" {
            n184 = call <vilib>:"Spark MAX Set Sensor Position.vi"("Position"=0.0, "MotorControlDeviceRef"=w419) -> ()  [unwired: 8 in, 2 out]
            n185 = local read item#?() -> (w424:dbl)
            n186 = call <vilib>:"WPI_RobotDriveTankDrive.vi"("Right axis value"=-0.5 ("Left axis value"), "Left axis value"=-0.5, "RobotDriveDevRef"=w422) -> ("RobotDriveDevRef"=w426:T5)  [unwired: 6 in, 2 out]
            n187 = call <vilib>:"Spark MAX Set Sensor Position.vi"("Position"=0.0) -> ()  [unwired: 9 in, 2 out]
            n188 = Less?(x=w424, y=-35.0) -> (x < y?=w425:bool)
            n189 = case shown="True" w425 {
              tunnel: w426 -> [_ w432]
              tunnel: w418 -> [_ w431]
              frame False {
              }
              frame True {
                n190 = call <vilib>:"WPI_RobotDriveTankDrive.vi"("Right axis value"=0.0 ("Left axis value"), "Left axis value"=0.0, "RobotDriveDevRef"=w432) -> ()  [unwired: 6 in, 3 out]
                n191 = call <vilib>:"Spark MAX Set Sensor Position.vi"("Position"=0.0, "MotorControlDeviceRef"=w431) -> ()  [unwired: 8 in, 2 out]
              }
            }
          }
        }
        n192 = Wait (ms)(milliseconds to wait=u32 20) -> ()  [unwired: 1 out]
      }
    }
    frame "blueesquerda" {
      n193 = call <vilib>:"WPI_RobotDriveRefNum Registry Get.vi"("refnum name"="rd") -> ("RobotDriveDevRef"=w439:T5)  [unwired: 9 in, 1 out]
      n194 = call <vilib>:"WPI_RobotDriveSafetyConfig.vi"("mode"=WPI_SafetyOutputConfigMenu."Enable", "RobotDriveDevRef"=w439) -> ("RobotDriveDevRef"=w435:T5)  [unwired: 8 in, 1 out]
      n195 = call <vilib>:"WPI_RobotDriveRefNum Registry Get.vi"("refnum name"="tracao") -> ("error out"=w461:errorcluster, "RobotDriveDevRef"=w460:T5)  [unwired: 9 in]
      n196 = call <vilib>:"WPI_RobotDriveSafetyConfig.vi"("error in (no error)"=w461, "mode"=WPI_SafetyOutputConfigMenu."Enable", "RobotDriveDevRef"=w460) -> ("RobotDriveDevRef"=w446:T5)  [unwired: 7 in, 1 out]
      n197 = Unbundle By Name(w435) -> ("Motors[]"=w445:T6[])
      n198 = Unbundle By Name(w446) -> ("Motors[]"=w458:T6[])
      n199 = Index Array(array=w458) -> (element #1=w450:T6, element #2=w453:T6, element #3=w452:T6, element #4=w451:T6)  [unwired: 4 in]
      n200 = Index Array(array=w445) -> (element #1=w442:T6, element #2=w443:T6)  [unwired: 2 in]
      n201 = call <vilib>:"Spark MAX Set Idle Mode.vi"("Idle Mode"=Spark_MAX_Idle_Mode."Brake", "MotorControlDeviceRef in"=w450) -> ()  [unwired: 8 in, 2 out]
      n202 = call <vilib>:"Spark MAX Set Idle Mode.vi"("Idle Mode"=Spark_MAX_Idle_Mode."Brake", "MotorControlDeviceRef in"=w453) -> ()  [unwired: 8 in, 2 out]
      n203 = call <vilib>:"Spark MAX Set Idle Mode.vi"("Idle Mode"=Spark_MAX_Idle_Mode."Brake", "MotorControlDeviceRef in"=w452) -> ()  [unwired: 8 in, 2 out]
      n204 = call <vilib>:"Spark MAX Set Idle Mode.vi"("Idle Mode"=Spark_MAX_Idle_Mode."Brake", "MotorControlDeviceRef in"=w451) -> ()  [unwired: 8 in, 2 out]
      n205 = call <vilib>:"Spark MAX Set Sensor Position.vi"("Position"=0.0, "MotorControlDeviceRef"=w450) -> ("MotorControlDeviceRef"=w448:T6)  [unwired: 8 in, 1 out]
      n206 = call <vilib>:"Spark MAX Set Sensor Position.vi"("Position"=0.0, "MotorControlDeviceRef"=w443) -> ("MotorControlDeviceRef"=w436:T6)  [unwired: 8 in, 1 out]
      n207 = call <vilib>:"Spark MAX Set Sensor Position.vi"("Position"=0.0, "MotorControlDeviceRef"=w442) -> ("MotorControlDeviceRef"=w437:T6)  [unwired: 8 in, 1 out]
      n208 = while {
        shift-right: [w471] -> _
        shift-left: T4."ação 1" -> [w476]
        tunnel: w448 -> [w474]
        tunnel: w446 -> [w472]
        tunnel: w437 -> [w469]
        tunnel: w436 -> [w468]
        tunnel: w435 -> [w465]
        stop <- w475 stop-if-true
        n209 = call <vilib>:"Spark MAX Get Sensor Position.vi"("MotorControlDevRef in"=w469) -> ("Sensor Position"=→"Sensor Position 12":dbl, "MotorControlDevRef out"=w464:T6)  [unwired: 7 in, 2 out]
        n210 = call <vilib>:"Spark MAX Get Sensor Position.vi"("MotorControlDevRef in"=w474) -> ("Sensor Position"=→"?":dbl, "MotorControlDevRef out"=w470:T6)  [unwired: 7 in, 2 out]
        n211 = call <vilib>:"Spark MAX Get Sensor Position.vi"("MotorControlDevRef in"=w468) -> ("Sensor Position"=→"Sensor Position 11":dbl, "MotorControlDevRef out"=w463:T6)  [unwired: 7 in, 2 out]
        n212 = case shown="\"ação 4\"" w476 {
          tunnel: [FALSE FALSE FALSE FALSE w544] -> w475
          tunnel: [w482 T4."ação 3" w507 w524 T4."ação 5"] -> w471
          tunnel: w472 -> [_ _ w509 w526 w541]
          tunnel: w470 -> [_ _ w506 w523 w536]
          tunnel: w465 -> [w478 w497 _ _ _]
          tunnel: w464 -> [_ _ w503 w520 w538]
          tunnel: w463 -> [_ _ w502 w519 w537]
          frame "ação 1", Default {
            n213 = local read "Sensor Position 11"() -> (w480:dbl)
            n214 = Greater?(x=w480, y=170.0) -> (0:w481:bool)
            n215 = call <vilib>:"WPI_RobotDriveTankDrive.vi"("Right axis value"=1.0, "Left axis value"=0.0, "RobotDriveDevRef"=w478) -> ("RobotDriveDevRef"=w484:T5)  [unwired: 6 in, 2 out]
            n216 = case shown="True" w481 {
              tunnel: w484 -> [_ w492]
              tunnel: [T4."ação 1" w488] -> w482
              frame False {
              }
              frame True {
                n217 = local read "Sensor Position 12"() -> (w490:dbl)
                n218 = call <vilib>:"WPI_RobotDriveTankDrive.vi"("Right axis value"=1.0 ("Left axis value"), "Left axis value"=1.0 ("Right axis value"), "RobotDriveDevRef"=w492) -> ()  [unwired: 6 in, 3 out]
                n219 = Greater?(x=w490, y=170.0) -> (0:w489:bool)
                n220 = case shown="False" w489 {
                  tunnel: [T4."ação 1" T4."ação 2"] -> w488
                  frame False {
                  }
                  frame True {
                  }
                }
              }
            }
          }
          frame "ação 2" {
            n221 = call <vilib>:"WPI_RobotDriveTankDrive.vi"("Right axis value"=0.0 ("Left axis value"), "Left axis value"=0.0, "RobotDriveDevRef"=w497) -> ()  [unwired: 6 in, 3 out]
          }
          frame "ação 3" {
            n222 = call <vilib>:"Spark MAX Set Sensor Position.vi"("Position"=0.0, "MotorControlDeviceRef"=w503) -> ()  [unwired: 8 in, 2 out]
            n223 = local read item#7() -> (w508:dbl)
            n224 = call <vilib>:"Spark MAX Set Sensor Position.vi"("Position"=0.0, "MotorControlDeviceRef"=w502) -> ()  [unwired: 8 in, 2 out]
            n225 = Greater?(x=w508, y=17.0) -> (0:w512:bool)
            n226 = call <vilib>:"WPI_RobotDriveTankDrive.vi"("Right axis value"=0.5 ("Left axis value"), "Left axis value"=0.5, "RobotDriveDevRef"=w509) -> ()  [unwired: 6 in, 3 out]
            n227 = case shown="True" w512 {
              tunnel: [T4."ação 3" T4."ação 4"] -> w507
              tunnel: w506 -> [_ w516]
              frame False {
              }
              frame True {
                n228 = call <vilib>:"Spark MAX Set Sensor Position.vi"("Position"=0.0, "MotorControlDeviceRef"=w516) -> ()  [unwired: 8 in, 2 out]
              }
            }
          }
          frame "ação 4" {
            n229 = call <vilib>:"Spark MAX Set Sensor Position.vi"("Position"=0.0, "MotorControlDeviceRef"=w520) -> ()  [unwired: 8 in, 2 out]
            n230 = local read item#7() -> (w525:dbl)
            n231 = call <vilib>:"Spark MAX Set Sensor Position.vi"("Position"=0.0, "MotorControlDeviceRef"=w519) -> ()  [unwired: 8 in, 2 out]
            n232 = call <vilib>:"WPI_RobotDriveTankDrive.vi"("Right axis value"=0.5 ("Left axis value"), "Left axis value"=-0.5, "RobotDriveDevRef"=w526) -> ()  [unwired: 6 in, 3 out]
            n233 = Less?(x=w525, y=-14.0) -> (x < y?=w528:bool)
            n234 = case shown="True" w528 {
              tunnel: [T4."ação 4" T4."ação 5"] -> w524
              tunnel: w523 -> [_ w533]
              frame False {
              }
              frame True {
                n235 = call <vilib>:"Spark MAX Set Sensor Position.vi"("Position"=0.0, "MotorControlDeviceRef"=w533) -> ()  [unwired: 8 in, 2 out]
              }
            }
          }
          frame "ação 5" {
            n236 = call <vilib>:"Spark MAX Set Sensor Position.vi"("Position"=0.0, "MotorControlDeviceRef"=w538) -> ()  [unwired: 8 in, 2 out]
            n237 = local read item#7() -> (w543:dbl)
            n238 = call <vilib>:"Spark MAX Set Sensor Position.vi"("Position"=0.0, "MotorControlDeviceRef"=w537) -> ()  [unwired: 8 in, 2 out]
            n239 = call <vilib>:"WPI_RobotDriveTankDrive.vi"("Right axis value"=-0.5 ("Left axis value"), "Left axis value"=-0.5, "RobotDriveDevRef"=w541) -> ("RobotDriveDevRef"=w545:T5)  [unwired: 6 in, 2 out]
            n240 = Less?(x=w543, y=-35.0) -> (x < y?=w544:bool)
            n241 = case shown="True" w544 {
              tunnel: w545 -> [_ w550]
              tunnel: w536 -> [_ w549]
              frame False {
              }
              frame True {
                n242 = call <vilib>:"WPI_RobotDriveTankDrive.vi"("Right axis value"=0.0 ("Left axis value"), "Left axis value"=0.0, "RobotDriveDevRef"=w550) -> ()  [unwired: 6 in, 3 out]
                n243 = call <vilib>:"Spark MAX Set Sensor Position.vi"("MotorControlDeviceRef"=w549) -> ()  [unwired: 9 in, 2 out]
              }
            }
          }
        }
        n244 = Wait (ms)(milliseconds to wait=u32 20) -> ()  [unwired: 1 out]
      }
    }
    frame "redmeiold" {
      n245 = call <vilib>:"WPI_RobotDriveRefNum Registry Get.vi"("refnum name"="tracao") -> ("error out"=w579:errorcluster, "RobotDriveDevRef"=w578:T5)  [unwired: 9 in]
      n246 = call <vilib>:"WPI_RobotDriveSafetyConfig.vi"("error in (no error)"=w579, "mode"=WPI_SafetyOutputConfigMenu."Enable", "RobotDriveDevRef"=w578) -> ("RobotDriveDevRef"=w569:T5)  [unwired: 7 in, 1 out]
      n247 = Unbundle By Name(w569) -> ("Motors[]"=w577:T6[])
      n248 = call <vilib>:"WPI_RobotDriveRefNum Registry Get.vi"("refnum name"="rd") -> ("RobotDriveDevRef"=w557:T5)  [unwired: 9 in, 1 out]
      n249 = call <vilib>:"WPI_RobotDriveSafetyConfig.vi"("mode"=WPI_SafetyOutputConfigMenu."Enable", "RobotDriveDevRef"=w557) -> ("RobotDriveDevRef"=w553:T5)  [unwired: 8 in, 1 out]
      n250 = Index Array(array=w577) -> (element #1=w570:T6, element #2=w574:T6, element #3=w573:T6, element #4=w572:T6)  [unwired: 4 in]
      n251 = call <vilib>:"Spark MAX Set Idle Mode.vi"("Idle Mode"=Spark_MAX_Idle_Mode."Brake", "MotorControlDeviceRef in"=w570) -> ()  [unwired: 8 in, 2 out]
      n252 = call <vilib>:"Spark MAX Set Idle Mode.vi"("Idle Mode"=Spark_MAX_Idle_Mode."Brake", "MotorControlDeviceRef in"=w574) -> ()  [unwired: 8 in, 2 out]
      n253 = call <vilib>:"Spark MAX Set Idle Mode.vi"("Idle Mode"=Spark_MAX_Idle_Mode."Brake", "MotorControlDeviceRef in"=w573) -> ()  [unwired: 8 in, 2 out]
      n254 = call <vilib>:"Spark MAX Set Idle Mode.vi"("Idle Mode"=Spark_MAX_Idle_Mode."Brake", "MotorControlDeviceRef in"=w572) -> ()  [unwired: 8 in, 2 out]
      n255 = Unbundle By Name(w553) -> ("Motors[]"=w563:T6[])
      n256 = call <vilib>:"Spark MAX Set Sensor Position.vi"("Position"=0.0, "MotorControlDeviceRef"=w570) -> ("MotorControlDeviceRef"=w568:T6)  [unwired: 8 in, 1 out]
      n257 = Index Array(array=w563) -> (element #1=w560:T6, element #2=w561:T6)  [unwired: 2 in]
      n258 = call <vilib>:"Spark MAX Set Sensor Position.vi"("Position"=0.0, "MotorControlDeviceRef"=w561) -> ("MotorControlDeviceRef"=w554:T6)  [unwired: 8 in, 1 out]
      n259 = call <vilib>:"Spark MAX Set Sensor Position.vi"("Position"=0.0, "MotorControlDeviceRef"=w560) -> ("MotorControlDeviceRef"=w555:T6)  [unwired: 8 in, 1 out]
      n260 = while {
        shift-right: [w593] -> _
        shift-left: T2."ação 1" -> [w594]
        tunnel: w569 -> [w592]
        tunnel: w568 -> [w590]
        tunnel: w555 -> [w587]
        tunnel: w554 -> [w586]
        tunnel: w553 -> [w583]
        stop <- w588 stop-if-true
        n261 = call <vilib>:"Spark MAX Get Sensor Position.vi"("MotorControlDevRef in"=w590) -> ("Sensor Position"=→"Sensor Position 2":dbl, "MotorControlDevRef out"=w589:T6)  [unwired: 7 in, 2 out]
        n262 = Wait (ms)(milliseconds to wait=u32 20) -> ()  [unwired: 1 out]
        n263 = call <vilib>:"Spark MAX Get Sensor Position.vi"("MotorControlDevRef in"=w587) -> ("Sensor Position"=→"Sensor Position 14":dbl, "MotorControlDevRef out"=w582:T6)  [unwired: 7 in, 2 out]
        n264 = call <vilib>:"Spark MAX Get Sensor Position.vi"("MotorControlDevRef in"=w586) -> ("Sensor Position"=→"Sensor Position 13":dbl, "MotorControlDevRef out"=w581:T6)  [unwired: 7 in, 2 out]
        n265 = case shown="\"ação 8\"" w594 {
          tunnel: [w601 T2."ação 3" w625 w642 w659 w677 T2."ação 8"] -> w593
          tunnel: w592 -> [_ _ w632 w649 w663 w683 w700]
          tunnel: w589 -> [_ _ w626 w643 w666 w678 w688]
          tunnel: [FALSE FALSE FALSE FALSE FALSE FALSE w694] -> w588
          tunnel: w583 -> [w596 w615 _ _ _ _ _]
          tunnel: w582 -> [_ _ w621 w638 w655 w672 w690]
          tunnel: w581 -> [_ _ w620 w637 w654 w671 w689]
          frame "ação 1", Default {
            n266 = local read "Sensor Position 13"() -> (w597:dbl)
            n267 = call <vilib>:"WPI_RobotDriveTankDrive.vi"("Right axis value"=1.0, "Left axis value"=0.0, "RobotDriveDevRef"=w596) -> ("RobotDriveDevRef"=w602:T5)  [unwired: 6 in, 2 out]
            n268 = Greater?(x=w597, y=150) -> (0:w598:bool)
            n269 = case shown="True" w598 {
              tunnel: w602 -> [_ w610]
              tunnel: [T2."ação 1" w608] -> w601
              frame False {
              }
              frame True {
                n270 = local read "Sensor Position 14"() -> (w607:dbl)
                n271 = call <vilib>:"WPI_RobotDriveTankDrive.vi"("Right axis value"=1.0 ("Left axis value"), "Left axis value"=1.0 ("Right axis value"), "RobotDriveDevRef"=w610) -> ()  [unwired: 6 in, 3 out]
                n272 = Greater?(x=w607, y=150.0) -> (0:w609:bool)
                n273 = case shown="True" w609 {
                  tunnel: [T2."ação 1" T2."ação 2"] -> w608
                  frame False {
                  }
                  frame True {
                  }
                }
              }
            }
          }
          frame "ação 2" {
            n274 = call <vilib>:"WPI_RobotDriveTankDrive.vi"("Right axis value"=0.0, "Left axis value"=0.0, "RobotDriveDevRef"=w615) -> ()  [unwired: 6 in, 3 out]
          }
          frame "ação 3" {
            n275 = local read "Sensor Position 2"() -> (w628:dbl)
            n276 = call <vilib>:"Spark MAX Set Sensor Position.vi"("Position"=0.0, "MotorControlDeviceRef"=w621) -> ()  [unwired: 8 in, 2 out]
            n277 = call <vilib>:"Spark MAX Set Sensor Position.vi"("Position"=0.0, "MotorControlDeviceRef"=w620) -> ()  [unwired: 8 in, 2 out]
            n278 = Greater?(x=w628, y=10.0) -> (0:w629:bool)
            n279 = call <vilib>:"WPI_RobotDriveTankDrive.vi"("Right axis value"=0.5 ("Left axis value"), "Left axis value"=0.5, "RobotDriveDevRef"=w632) -> ()  [unwired: 6 in, 3 out]
            n280 = case shown="True" w629 {
              tunnel: w626 -> [_ w636]
              tunnel: [T2."ação 3" T2."ação 4"] -> w625
              frame False {
              }
              frame True {
                n281 = call <vilib>:"Spark MAX Set Sensor Position.vi"("Position"=0.0, "MotorControlDeviceRef"=w636) -> ()  [unwired: 8 in, 2 out]
              }
            }
          }
          frame "ação 4" {
            n282 = local read "Sensor Position 2"() -> (w646:dbl)
            n283 = call <vilib>:"Spark MAX Set Sensor Position.vi"("Position"=0.0, "MotorControlDeviceRef"=w638) -> ()  [unwired: 8 in, 2 out]
            n284 = call <vilib>:"Spark MAX Set Sensor Position.vi"("Position"=0.0, "MotorControlDeviceRef"=w637) -> ()  [unwired: 8 in, 2 out]
            n285 = call <vilib>:"WPI_RobotDriveTankDrive.vi"("Right axis value"=0.5 ("Left axis value"), "Left axis value"=-0.5, "RobotDriveDevRef"=w649) -> ()  [unwired: 6 in, 3 out]
            n286 = Less?(x=w646, y=-6.0) -> (x < y?=w644:bool)
            n287 = case shown="True" w644 {
              tunnel: w643 -> [_ w653]
              tunnel: [T2."ação 4" T2."ação 5"] -> w642
              frame False {
              }
              frame True {
                n288 = call <vilib>:"Spark MAX Set Sensor Position.vi"("Position"=0.0, "MotorControlDeviceRef"=w653) -> ()  [unwired: 8 in, 2 out]
              }
            }
          }
          frame "ação 5" {
            n289 = local read "Sensor Position 2"() -> (w662:dbl)
            n290 = call <vilib>:"Spark MAX Set Sensor Position.vi"("Position"=0.0, "MotorControlDeviceRef"=w655) -> ()  [unwired: 8 in, 2 out]
            n291 = call <vilib>:"WPI_RobotDriveTankDrive.vi"("Right axis value"=-0.5 ("Left axis value"), "Left axis value"=-0.5, "RobotDriveDevRef"=w663) -> ()  [unwired: 6 in, 3 out]
            n292 = call <vilib>:"Spark MAX Set Sensor Position.vi"("Position"=0.0, "MotorControlDeviceRef"=w654) -> ()  [unwired: 8 in, 2 out]
            n293 = Less?(x=w662, y=-13.0) -> (x < y?=w660:bool)
            n294 = case shown="True" w660 {
              tunnel: w666 -> [_ w669]
              tunnel: [T2."ação 5" T2."ação 7"] -> w659
              frame False {
              }
              frame True {
                n295 = call <vilib>:"Spark MAX Set Sensor Position.vi"("Position"=0.0, "MotorControlDeviceRef"=w669) -> ()  [unwired: 8 in, 2 out]
              }
            }
          }
          frame "ação 7" {
            n296 = local read "Sensor Position 2"() -> (w680:dbl)
            n297 = call <vilib>:"Spark MAX Set Sensor Position.vi"("Position"=0.0, "MotorControlDeviceRef"=w672) -> ()  [unwired: 8 in, 2 out]
            n298 = call <vilib>:"WPI_RobotDriveTankDrive.vi"("Right axis value"=0.5 ("Left axis value"), "Left axis value"=-0.5, "RobotDriveDevRef"=w683) -> ()  [unwired: 6 in, 3 out]
            n299 = call <vilib>:"Spark MAX Set Sensor Position.vi"("Position"=0.0, "MotorControlDeviceRef"=w671) -> ()  [unwired: 8 in, 2 out]
            n300 = Less?(x=w680, y=-8.3) -> (x < y?=w679:bool)
            n301 = case shown="True" w679 {
              tunnel: w678 -> [_ w687]
              tunnel: [T2."ação 7" T2."ação 8"] -> w677
              frame False {
              }
              frame True {
                n302 = call <vilib>:"Spark MAX Set Sensor Position.vi"("Position"=0.0, "MotorControlDeviceRef"=w687) -> ()  [unwired: 8 in, 2 out]
              }
            }
          }
          frame "ação 8" {
            n303 = local read "Sensor Position 2"() -> (w697:dbl)
            n304 = call <vilib>:"Spark MAX Set Sensor Position.vi"("Position"=0.0, "MotorControlDeviceRef"=w690) -> ()  [unwired: 8 in, 2 out]
            n305 = call <vilib>:"WPI_RobotDriveTankDrive.vi"("Right axis value"=-0.5 ("Left axis value"), "Left axis value"=-0.5, "RobotDriveDevRef"=w700) -> ("RobotDriveDevRef"=w695:T5)  [unwired: 6 in, 2 out]
            n306 = call <vilib>:"Spark MAX Set Sensor Position.vi"("Position"=0.0, "MotorControlDeviceRef"=w689) -> ()  [unwired: 8 in, 2 out]
            n307 = Less?(x=w697, y=-45.0) -> (x < y?=w694:bool)
            n308 = case shown="True" w694 {
              tunnel: w695 -> [_ w705]
              tunnel: w688 -> [_ w702]
              frame False {
              }
              frame True {
                n309 = call <vilib>:"WPI_RobotDriveTankDrive.vi"("Right axis value"=0.0 ("Left axis value"), "Left axis value"=0.0, "RobotDriveDevRef"=w705) -> ()  [unwired: 6 in, 3 out]
                n310 = call <vilib>:"Spark MAX Set Sensor Position.vi"("Position"=0.0, "MotorControlDeviceRef"=w702) -> ()  [unwired: 8 in, 2 out]
              }
            }
          }
        }
      }
    }
    frame "bluemeiole" {
      n311 = call <vilib>:"WPI_RobotDriveRefNum Registry Get.vi"("refnum name"="tracao") -> ("error out"=w732:errorcluster, "RobotDriveDevRef"=w731:T5)  [unwired: 9 in]
      n312 = call <vilib>:"WPI_RobotDriveSafetyConfig.vi"("error in (no error)"=w732, "mode"=WPI_SafetyOutputConfigMenu."Enable", "RobotDriveDevRef"=w731) -> ("RobotDriveDevRef"=w722:T5)  [unwired: 7 in, 1 out]
      n313 = Unbundle By Name(w722) -> ("Motors[]"=w730:T6[])
      n314 = call <vilib>:"WPI_RobotDriveRefNum Registry Get.vi"("refnum name"="rd") -> ("RobotDriveDevRef"=w710:T5)  [unwired: 9 in, 1 out]
      n315 = Index Array(array=w730) -> (element #1=w723:T6, element #2=w727:T6, element #3=w726:T6, element #4=w725:T6)  [unwired: 4 in]
      n316 = call <vilib>:"WPI_RobotDriveSafetyConfig.vi"("mode"=WPI_SafetyOutputConfigMenu."Enable", "RobotDriveDevRef"=w710) -> ("RobotDriveDevRef"=w706:T5)  [unwired: 8 in, 1 out]
      n317 = call <vilib>:"Spark MAX Set Idle Mode.vi"("Idle Mode"=Spark_MAX_Idle_Mode."Brake", "MotorControlDeviceRef in"=w723) -> ()  [unwired: 8 in, 2 out]
      n318 = call <vilib>:"Spark MAX Set Idle Mode.vi"("Idle Mode"=Spark_MAX_Idle_Mode."Brake", "MotorControlDeviceRef in"=w727) -> ()  [unwired: 8 in, 2 out]
      n319 = call <vilib>:"Spark MAX Set Idle Mode.vi"("Idle Mode"=Spark_MAX_Idle_Mode."Brake", "MotorControlDeviceRef in"=w726) -> ()  [unwired: 8 in, 2 out]
      n320 = call <vilib>:"Spark MAX Set Idle Mode.vi"("Idle Mode"=Spark_MAX_Idle_Mode."Brake", "MotorControlDeviceRef in"=w725) -> ()  [unwired: 8 in, 2 out]
      n321 = call <vilib>:"Spark MAX Set Sensor Position.vi"("Position"=0.0, "MotorControlDeviceRef"=w723) -> ("MotorControlDeviceRef"=w721:T6)  [unwired: 8 in, 1 out]
      n322 = Unbundle By Name(w706) -> ("Motors[]"=w716:T6[])
      n323 = Index Array(array=w716) -> (element #1=w713:T6, element #2=w714:T6)  [unwired: 2 in]
      n324 = call <vilib>:"Spark MAX Set Sensor Position.vi"("Position"=0.0, "MotorControlDeviceRef"=w714) -> ("MotorControlDeviceRef"=w707:T6)  [unwired: 8 in, 1 out]
      n325 = call <vilib>:"Spark MAX Set Sensor Position.vi"("Position"=0.0, "MotorControlDeviceRef"=w713) -> ("MotorControlDeviceRef"=w708:T6)  [unwired: 8 in, 1 out]
      n326 = while {
        shift-right: [w746] -> _
        shift-left: T2."ação 1" -> [w747]
        tunnel: w722 -> [w745]
        tunnel: w721 -> [w743]
        tunnel: w708 -> [w740]
        tunnel: w707 -> [w739]
        tunnel: w706 -> [w736]
        stop <- w741 stop-if-true
        n327 = call <vilib>:"Spark MAX Get Sensor Position.vi"("MotorControlDevRef in"=w740) -> ("Sensor Position"=→"Sensor Position 15":dbl, "MotorControlDevRef out"=w735:T6)  [unwired: 7 in, 2 out]
        n328 = call <vilib>:"Spark MAX Get Sensor Position.vi"("MotorControlDevRef in"=w739) -> ("Sensor Position"=→"Sensor Position 16":dbl, "MotorControlDevRef out"=w734:T6)  [unwired: 7 in, 2 out]
        n329 = call <vilib>:"Spark MAX Get Sensor Position.vi"("MotorControlDevRef in"=w743) -> ("Sensor Position"=→"Sensor Position 5":dbl, "MotorControlDevRef out"=w742:T6)  [unwired: 7 in, 2 out]
        n330 = case shown="\"ação 8\"" w747 {
          tunnel: [w752 T2."ação 3" w778 w795 w812 w829 T2."ação 8"] -> w746
          tunnel: w745 -> [_ _ w785 w802 w816 w836 w853]
          tunnel: w742 -> [_ _ w779 w796 w819 w830 w841]
          tunnel: [FALSE FALSE FALSE FALSE FALSE FALSE w847] -> w741
          tunnel: w736 -> [w749 w768 _ _ _ _ _]
          tunnel: w735 -> [_ _ w774 w790 w807 w824 w842]
          tunnel: w734 -> [_ _ w773 w791 w808 w825 w843]
          frame "ação 1", Default {
            n331 = local read "Sensor Position 16"() -> (w750:dbl)
            n332 = call <vilib>:"WPI_RobotDriveTankDrive.vi"("Right axis value"=1.0, "Left axis value"=0.0, "RobotDriveDevRef"=w749) -> ("RobotDriveDevRef"=w755:T5)  [unwired: 6 in, 2 out]
            n333 = Greater?(x=w750, y=u32 150) -> (0:w753:bool)
            n334 = case shown="True" w753 {
              tunnel: w755 -> [_ w763]
              tunnel: [T2."ação 1" w759] -> w752
              frame False {
              }
              frame True {
                n335 = local read "Sensor Position 15"() -> (w762:dbl)
                n336 = Greater?(x=w762, y=150.0) -> (0:w760:bool)
                n337 = call <vilib>:"WPI_RobotDriveTankDrive.vi"("Right axis value"=1.0 ("Left axis value"), "Left axis value"=1.0 ("Right axis value"), "RobotDriveDevRef"=w763) -> ()  [unwired: 6 in, 3 out]
                n338 = case shown="False" w760 {
                  tunnel: [T2."ação 1" T2."ação 2"] -> w759
                  frame False {
                  }
                  frame True {
                  }
                }
              }
            }
          }
          frame "ação 2" {
            n339 = call <vilib>:"WPI_RobotDriveTankDrive.vi"("Right axis value"=0.0, "Left axis value"=0.0, "RobotDriveDevRef"=w768) -> ()  [unwired: 6 in, 3 out]
          }
          frame "ação 3" {
            n340 = local read "Sensor Position 5"() -> (w781:dbl)
            n341 = call <vilib>:"Spark MAX Set Sensor Position.vi"("Position"=0.0, "MotorControlDeviceRef"=w774) -> ()  [unwired: 8 in, 2 out]
            n342 = call <vilib>:"Spark MAX Set Sensor Position.vi"("Position"=0.0, "MotorControlDeviceRef"=w773) -> ()  [unwired: 8 in, 2 out]
            n343 = Greater?(x=w781, y=10.0) -> (0:w782:bool)
            n344 = call <vilib>:"WPI_RobotDriveTankDrive.vi"("Right axis value"=0.5 ("Left axis value"), "Left axis value"=0.5, "RobotDriveDevRef"=w785) -> ()  [unwired: 6 in, 3 out]
            n345 = case shown="True" w782 {
              tunnel: w779 -> [_ w789]
              tunnel: [T2."ação 3" T2."ação 4"] -> w778
              frame False {
              }
              frame True {
                n346 = call <vilib>:"Spark MAX Set Sensor Position.vi"("Position"=0.0, "MotorControlDeviceRef"=w789) -> ()  [unwired: 8 in, 2 out]
              }
            }
          }
          frame "ação 4" {
            n347 = local read "Sensor Position 5"() -> (w799:dbl)
            n348 = call <vilib>:"Spark MAX Set Sensor Position.vi"("Position"=0.0, "MotorControlDeviceRef"=w791) -> ()  [unwired: 8 in, 2 out]
            n349 = call <vilib>:"Spark MAX Set Sensor Position.vi"("Position"=0.0, "MotorControlDeviceRef"=w790) -> ()  [unwired: 8 in, 2 out]
            n350 = call <vilib>:"WPI_RobotDriveTankDrive.vi"("Right axis value"=-0.5 ("Left axis value"), "Left axis value"=0.5, "RobotDriveDevRef"=w802) -> ()  [unwired: 6 in, 3 out]
            n351 = Greater?(x=w799, y=6.0) -> (0:w797:bool)
            n352 = case shown="True" w797 {
              tunnel: w796 -> [_ w806]
              tunnel: [T2."ação 4" T2."ação 5"] -> w795
              frame False {
              }
              frame True {
                n353 = call <vilib>:"Spark MAX Set Sensor Position.vi"("Position"=0.0, "MotorControlDeviceRef"=w806) -> ()  [unwired: 8 in, 2 out]
              }
            }
          }
          frame "ação 5" {
            n354 = local read "Sensor Position 5"() -> (w815:dbl)
            n355 = call <vilib>:"Spark MAX Set Sensor Position.vi"("Position"=0.0, "MotorControlDeviceRef"=w808) -> ()  [unwired: 8 in, 2 out]
            n356 = call <vilib>:"WPI_RobotDriveTankDrive.vi"("Right axis value"=-0.5 ("Left axis value"), "Left axis value"=-0.5, "RobotDriveDevRef"=w816) -> ()  [unwired: 6 in, 3 out]
            n357 = call <vilib>:"Spark MAX Set Sensor Position.vi"("Position"=0.0, "MotorControlDeviceRef"=w807) -> ()  [unwired: 8 in, 2 out]
            n358 = Less?(x=w815, y=-13.0) -> (x < y?=w813:bool)
            n359 = case shown="True" w813 {
              tunnel: w819 -> [_ w822]
              tunnel: [T2."ação 5" T2."ação 7"] -> w812
              frame False {
              }
              frame True {
                n360 = call <vilib>:"Spark MAX Set Sensor Position.vi"("Position"=0.0, "MotorControlDeviceRef"=w822) -> ()  [unwired: 8 in, 2 out]
              }
            }
          }
          frame "ação 7" {
            n361 = local read "Sensor Position 5"() -> (w833:dbl)
            n362 = call <vilib>:"Spark MAX Set Sensor Position.vi"("Position"=0.0, "MotorControlDeviceRef"=w825) -> ()  [unwired: 8 in, 2 out]
            n363 = call <vilib>:"WPI_RobotDriveTankDrive.vi"("Right axis value"=-0.5 ("Left axis value"), "Left axis value"=0.5, "RobotDriveDevRef"=w836) -> ()  [unwired: 6 in, 3 out]
            n364 = call <vilib>:"Spark MAX Set Sensor Position.vi"("Position"=0.0, "MotorControlDeviceRef"=w824) -> ()  [unwired: 8 in, 2 out]
            n365 = Greater?(x=w833, y=8.3) -> (0:w831:bool)
            n366 = case shown="True" w831 {
              tunnel: w830 -> [_ w840]
              tunnel: [T2."ação 7" T2."ação 8"] -> w829
              frame False {
              }
              frame True {
                n367 = call <vilib>:"Spark MAX Set Sensor Position.vi"("Position"=0.0, "MotorControlDeviceRef"=w840) -> ()  [unwired: 8 in, 2 out]
              }
            }
          }
          frame "ação 8" {
            n368 = local read "Sensor Position 5"() -> (w850:dbl)
            n369 = call <vilib>:"Spark MAX Set Sensor Position.vi"("Position"=0.0, "MotorControlDeviceRef"=w843) -> ()  [unwired: 8 in, 2 out]
            n370 = call <vilib>:"WPI_RobotDriveTankDrive.vi"("Right axis value"=-0.5 ("Left axis value"), "Left axis value"=-0.5, "RobotDriveDevRef"=w853) -> ("RobotDriveDevRef"=w848:T5)  [unwired: 6 in, 2 out]
            n371 = call <vilib>:"Spark MAX Set Sensor Position.vi"("Position"=0.0, "MotorControlDeviceRef"=w842) -> ()  [unwired: 8 in, 2 out]
            n372 = Less?(x=w850, y=-45.0) -> (x < y?=w847:bool)
            n373 = case shown="True" w847 {
              tunnel: w848 -> [_ w858]
              tunnel: w841 -> [_ w855]
              frame False {
              }
              frame True {
                n374 = call <vilib>:"WPI_RobotDriveTankDrive.vi"("Right axis value"=0.0 ("Left axis value"), "Left axis value"=0.0, "RobotDriveDevRef"=w858) -> ()  [unwired: 6 in, 3 out]
                n375 = call <vilib>:"Spark MAX Set Sensor Position.vi"("Position"=0.0, "MotorControlDeviceRef"=w855) -> ()  [unwired: 8 in, 2 out]
              }
            }
          }
        }
        n376 = Wait (ms)(milliseconds to wait=u32 20) -> ()  [unwired: 1 out]
      }
    }
    frame "redesquerda" {
      n377 = call <vilib>:"WPI_RobotDriveRefNum Registry Get.vi"("refnum name"="tracao") -> ("error out"=w885:errorcluster, "RobotDriveDevRef"=w884:T5)  [unwired: 9 in]
      n378 = call <vilib>:"WPI_RobotDriveSafetyConfig.vi"("error in (no error)"=w885, "mode"=WPI_SafetyOutputConfigMenu."Enable", "RobotDriveDevRef"=w884) -> ("RobotDriveDevRef"=w876:T5)  [unwired: 7 in, 1 out]
      n379 = call <vilib>:"WPI_RobotDriveRefNum Registry Get.vi"("refnum name"="rd") -> ("RobotDriveDevRef"=w864:T5)  [unwired: 9 in, 1 out]
      n380 = Unbundle By Name(w876) -> ("Motors[]"=w883:T6[])
      n381 = call <vilib>:"WPI_RobotDriveSafetyConfig.vi"("mode"=WPI_SafetyOutputConfigMenu."Enable", "RobotDriveDevRef"=w864) -> ("RobotDriveDevRef"=w860:T5)  [unwired: 8 in, 1 out]
      n382 = Index Array(array=w883) -> (element #1=w877:T6, element #2=w881:T6, element #3=w880:T6, element #4=w879:T6)  [unwired: 4 in]
      n383 = call <vilib>:"Spark MAX Set Idle Mode.vi"("Idle Mode"=Spark_MAX_Idle_Mode."Brake", "MotorControlDeviceRef in"=w877) -> ()  [unwired: 8 in, 2 out]
      n384 = call <vilib>:"Spark MAX Set Idle Mode.vi"("Idle Mode"=Spark_MAX_Idle_Mode."Brake", "MotorControlDeviceRef in"=w881) -> ()  [unwired: 8 in, 2 out]
      n385 = call <vilib>:"Spark MAX Set Idle Mode.vi"("Idle Mode"=Spark_MAX_Idle_Mode."Brake", "MotorControlDeviceRef in"=w880) -> ()  [unwired: 8 in, 2 out]
      n386 = call <vilib>:"Spark MAX Set Idle Mode.vi"("Idle Mode"=Spark_MAX_Idle_Mode."Brake", "MotorControlDeviceRef in"=w879) -> ()  [unwired: 8 in, 2 out]
      n387 = Unbundle By Name(w860) -> ("Motors[]"=w869:T6[])
      n388 = call <vilib>:"Spark MAX Set Sensor Position.vi"("Position"=0.0, "MotorControlDeviceRef"=w877) -> ("MotorControlDeviceRef"=w875:T6)  [unwired: 8 in, 1 out]
      n389 = Index Array(array=w869) -> (element #1=w866:T6, element #2=w867:T6)  [unwired: 2 in]
      n390 = call <vilib>:"Spark MAX Set Sensor Position.vi"("Position"=0.0, "MotorControlDeviceRef"=w867) -> ("MotorControlDeviceRef"=w861:T6)  [unwired: 8 in, 1 out]
      n391 = call <vilib>:"Spark MAX Set Sensor Position.vi"("Position"=0.0, "MotorControlDeviceRef"=w866) -> ("MotorControlDeviceRef"=w862:T6)  [unwired: 8 in, 1 out]
      n392 = while {
        shift-right: [w894] -> _
        shift-left: T4."ação 1" -> [w895]
        tunnel: w876 -> [w900]
        tunnel: w875 -> [w898]
        tunnel: w862 -> [w893]
        tunnel: w861 -> [w892]
        tunnel: w860 -> [w889]
        stop <- w896 stop-if-true
        n393 = call <vilib>:"Spark MAX Get Sensor Position.vi"("MotorControlDevRef in"=w898) -> ("Sensor Position"=→"Sensor Position 3":dbl, "MotorControlDevRef out"=w897:T6)  [unwired: 7 in, 2 out]
        n394 = call <vilib>:"Spark MAX Get Sensor Position.vi"("MotorControlDevRef in"=w893) -> ("Sensor Position"=→"Sensor Position 18":dbl, "MotorControlDevRef out"=w888:T6)  [unwired: 7 in, 2 out]
        n395 = call <vilib>:"Spark MAX Get Sensor Position.vi"("MotorControlDevRef in"=w892) -> ("Sensor Position"=→"Sensor Position 17":dbl, "MotorControlDevRef out"=w887:T6)  [unwired: 7 in, 2 out]
        n396 = case shown="\"ação 4\"" w895 {
          tunnel: w900 -> [_ _ w941 w958 w973]
          tunnel: w897 -> [w902 _ w935 w952 w963]
          tunnel: [FALSE FALSE FALSE FALSE w968] -> w896
          tunnel: [w908 T4."ação 3" w933 w950 T4."ação 5"] -> w894
          tunnel: w889 -> [w903 w924 _ _ _]
          tunnel: w888 -> [_ _ w930 w946 w965]
          tunnel: w887 -> [_ _ w929 w947 w964]
          frame "ação 1", Default {
            n397 = local read "Sensor Position 17"() -> (w904:dbl)
            n398 = call <vilib>:"WPI_RobotDriveTankDrive.vi"("Right axis value"=1.0, "Left axis value"=0.0, "RobotDriveDevRef"=w903) -> ("RobotDriveDevRef"=w907:T5)  [unwired: 6 in, 2 out]
            n399 = Greater?(x=w904, y=u32 150) -> (0:w905:bool)
            n400 = case shown="True" w905 {
              tunnel: w907 -> [_ w919]
              tunnel: [T4."ação 1" w916] -> w908
              tunnel: w902 -> [_ w913]
              frame False {
              }
              frame True {
                n401 = local read "Sensor Position 18"() -> (w918:dbl)
                n402 = call <vilib>:"Spark MAX Set Sensor Position.vi"("Position"=0.0, "MotorControlDeviceRef"=w913) -> ()  [unwired: 8 in, 2 out]
                n403 = call <vilib>:"WPI_RobotDriveTankDrive.vi"("Right axis value"=1.0 ("Left axis value"), "Left axis value"=1.0 ("Right axis value"), "RobotDriveDevRef"=w919) -> ()  [unwired: 6 in, 3 out]
                n404 = Greater?(x=w918, y=150.0) -> (0:w917:bool)
                n405 = case shown="False" w917 {
                  tunnel: [T4."ação 1" T4."ação 2"] -> w916
                  frame False {
                  }
                  frame True {
                  }
                }
              }
            }
          }
          frame "ação 2" {
            n406 = call <vilib>:"WPI_RobotDriveTankDrive.vi"("Right axis value"=0.0, "Left axis value"=0.0, "RobotDriveDevRef"=w924) -> ()  [unwired: 6 in, 3 out]
          }
          frame "ação 3" {
            n407 = local read "Sensor Position 3"() -> (w937:dbl)
            n408 = call <vilib>:"Spark MAX Set Sensor Position.vi"("Position"=0.0, "MotorControlDeviceRef"=w930) -> ()  [unwired: 8 in, 2 out]
            n409 = call <vilib>:"Spark MAX Set Sensor Position.vi"("Position"=0.0, "MotorControlDeviceRef"=w929) -> ()  [unwired: 8 in, 2 out]
            n410 = Greater?(x=w937, y=57.0) -> (0:w938:bool)
            n411 = call <vilib>:"WPI_RobotDriveTankDrive.vi"("Right axis value"=0.5 ("Left axis value"), "Left axis value"=0.5, "RobotDriveDevRef"=w941) -> ()  [unwired: 6 in, 3 out]
            n412 = case shown="True" w938 {
              tunnel: w935 -> [_ w945]
              tunnel: [T4."ação 3" T4."ação 4"] -> w933
              frame False {
              }
              frame True {
                n413 = call <vilib>:"Spark MAX Set Sensor Position.vi"("Position"=0.0, "MotorControlDeviceRef"=w945) -> ()  [unwired: 8 in, 2 out]
              }
            }
          }
          frame "ação 4" {
            n414 = local read "Sensor Position 3"() -> (w955:dbl)
            n415 = call <vilib>:"Spark MAX Set Sensor Position.vi"("Position"=0.0, "MotorControlDeviceRef"=w946) -> ()  [unwired: 8 in, 2 out]
            n416 = call <vilib>:"Spark MAX Set Sensor Position.vi"("Position"=0.0, "MotorControlDeviceRef"=w947) -> ()  [unwired: 8 in, 2 out]
            n417 = call <vilib>:"WPI_RobotDriveTankDrive.vi"("Right axis value"=0.5 ("Left axis value"), "Left axis value"=-0.5, "RobotDriveDevRef"=w958) -> ()  [unwired: 6 in, 3 out]
            n418 = Less?(x=w955, y=-14.0) -> (x < y?=w953:bool)
            n419 = case shown="True" w953 {
              tunnel: w952 -> [_ w962]
              tunnel: [T4."ação 4" T4."ação 5"] -> w950
              frame False {
              }
              frame True {
                n420 = call <vilib>:"Spark MAX Set Sensor Position.vi"("Position"=0.0, "MotorControlDeviceRef"=w962) -> ()  [unwired: 8 in, 2 out]
              }
            }
          }
          frame "ação 5" {
            n421 = local read "Sensor Position 3"() -> (w972:dbl)
            n422 = call <vilib>:"Spark MAX Set Sensor Position.vi"("Position"=0.0, "MotorControlDeviceRef"=w965) -> ()  [unwired: 8 in, 2 out]
            n423 = call <vilib>:"WPI_RobotDriveTankDrive.vi"("Right axis value"=-0.5 ("Left axis value"), "Left axis value"=-0.5, "RobotDriveDevRef"=w973) -> ("RobotDriveDevRef"=w970:T5)  [unwired: 6 in, 2 out]
            n424 = call <vilib>:"Spark MAX Set Sensor Position.vi"("Position"=0.0, "MotorControlDeviceRef"=w964) -> ()  [unwired: 8 in, 2 out]
            n425 = Less?(x=w972, y=-50.0) -> (x < y?=w968:bool)
            n426 = case shown="True" w968 {
              tunnel: w970 -> [_ w978]
              tunnel: w963 -> [_ w976]
              frame False {
              }
              frame True {
                n427 = call <vilib>:"WPI_RobotDriveTankDrive.vi"("Right axis value"=0.0 ("Left axis value"), "Left axis value"=0.0, "RobotDriveDevRef"=w978) -> ()  [unwired: 6 in, 3 out]
                n428 = call <vilib>:"Spark MAX Set Sensor Position.vi"("Position"=0.0, "MotorControlDeviceRef"=w976) -> ()  [unwired: 8 in, 2 out]
              }
            }
          }
        }
        n429 = Wait (ms)(milliseconds to wait=u32 20) -> ()  [unwired: 1 out]
      }
    }
    frame "bluedireita" {
      n430 = call <vilib>:"WPI_RobotDriveRefNum Registry Get.vi"("refnum name"="tracao") -> ("error out"=w1007:errorcluster, "RobotDriveDevRef"=w1006:T5)  [unwired: 9 in]
      n431 = call <vilib>:"WPI_RobotDriveRefNum Registry Get.vi"("refnum name"="rd") -> ("RobotDriveDevRef"=w986:T5)  [unwired: 9 in, 1 out]
      n432 = call <vilib>:"WPI_RobotDriveSafetyConfig.vi"("error in (no error)"=w1007, "mode"=WPI_SafetyOutputConfigMenu."Enable", "RobotDriveDevRef"=w1006) -> ("RobotDriveDevRef"=w998:T5)  [unwired: 7 in, 1 out]
      n433 = call <vilib>:"WPI_RobotDriveSafetyConfig.vi"("mode"=WPI_SafetyOutputConfigMenu."Enable", "RobotDriveDevRef"=w986) -> ("RobotDriveDevRef"=w982:T5)  [unwired: 8 in, 1 out]
      n434 = Unbundle By Name(w998) -> ("Motors[]"=w1005:T6[])
      n435 = Index Array(array=w1005) -> (element #1=w999:T6, element #2=w1003:T6, element #3=w1002:T6, element #4=w1001:T6)  [unwired: 4 in]
      n436 = Unbundle By Name(w982) -> ("Motors[]"=w991:T6[])
      n437 = call <vilib>:"Spark MAX Set Idle Mode.vi"("Idle Mode"=Spark_MAX_Idle_Mode."Brake", "MotorControlDeviceRef in"=w999) -> ()  [unwired: 8 in, 2 out]
      n438 = call <vilib>:"Spark MAX Set Idle Mode.vi"("Idle Mode"=Spark_MAX_Idle_Mode."Brake", "MotorControlDeviceRef in"=w1003) -> ()  [unwired: 8 in, 2 out]
      n439 = call <vilib>:"Spark MAX Set Idle Mode.vi"("Idle Mode"=Spark_MAX_Idle_Mode."Brake", "MotorControlDeviceRef in"=w1002) -> ()  [unwired: 8 in, 2 out]
      n440 = call <vilib>:"Spark MAX Set Idle Mode.vi"("Idle Mode"=Spark_MAX_Idle_Mode."Brake", "MotorControlDeviceRef in"=w1001) -> ()  [unwired: 8 in, 2 out]
      n441 = call <vilib>:"Spark MAX Set Sensor Position.vi"("Position"=0.0, "MotorControlDeviceRef"=w999) -> ("MotorControlDeviceRef"=w997:T6)  [unwired: 8 in, 1 out]
      n442 = Index Array(array=w991) -> (element #1=w988:T6, element #2=w989:T6)  [unwired: 2 in]
      n443 = call <vilib>:"Spark MAX Set Sensor Position.vi"("Position"=0.0, "MotorControlDeviceRef"=w989) -> ("MotorControlDeviceRef"=w983:T6)  [unwired: 8 in, 1 out]
      n444 = call <vilib>:"Spark MAX Set Sensor Position.vi"("Position"=0.0, "MotorControlDeviceRef"=w988) -> ("MotorControlDeviceRef"=w984:T6)  [unwired: 8 in, 1 out]
      n445 = while {
        shift-right: [w1016] -> _
        shift-left: T4."ação 1" -> [w1017]
        tunnel: w998 -> [w1022]
        tunnel: w997 -> [w1020]
        tunnel: w984 -> [w1015]
        tunnel: w983 -> [w1014]
        tunnel: w982 -> [w1011]
        stop <- w1018 stop-if-true
        n446 = call <vilib>:"Spark MAX Get Sensor Position.vi"("MotorControlDevRef in"=w1020) -> ("Sensor Position"=→"Sensor Position 4":dbl, "MotorControlDevRef out"=w1019:T6)  [unwired: 7 in, 2 out]
        n447 = call <vilib>:"Spark MAX Get Sensor Position.vi"("MotorControlDevRef in"=w1015) -> ("Sensor Position"=→"Sensor Position 19":dbl, "MotorControlDevRef out"=w1010:T6)  [unwired: 7 in, 2 out]
        n448 = Wait (ms)(milliseconds to wait=u32 20) -> ()  [unwired: 1 out]
        n449 = call <vilib>:"Spark MAX Get Sensor Position.vi"("MotorControlDevRef in"=w1014) -> ("Sensor Position"=→"Sensor Position 20":dbl, "MotorControlDevRef out"=w1009:T6)  [unwired: 7 in, 2 out]
        n450 = case shown="\"ação 4\"" w1017 {
          tunnel: w1022 -> [_ w1043 w1060 w1077 w1091]
          tunnel: w1019 -> [_ _ w1054 w1071 _]
          tunnel: [FALSE FALSE FALSE FALSE w1086] -> w1018
          tunnel: [w1026 T4."ação 3" w1052 w1069 T4."ação 5"] -> w1016
          tunnel: w1011 -> [w1024 _ _ _ _]
          tunnel: w1010 -> [_ _ w1049 w1065 w1083]
          tunnel: w1009 -> [_ _ w1048 w1066 w1082]
          frame "ação 1", Default {
            n451 = local read "Sensor Position 20"() -> (w1025:dbl)
            n452 = call <vilib>:"WPI_RobotDriveTankDrive.vi"("Right axis value"=1.0, "Left axis value"=0.0, "RobotDriveDevRef"=w1024) -> ("RobotDriveDevRef"=w1030:T5)  [unwired: 6 in, 2 out]
            n453 = Greater?(x=w1025, y=u32 170) -> (0:w1028:bool)
            n454 = case shown="True" w1028 {
              tunnel: w1030 -> [_ w1038]
              tunnel: [T4."ação 1" w1034] -> w1026
              frame False {
              }
              frame True {
                n455 = local read "Sensor Position 19"() -> (w1037:dbl)
                n456 = call <vilib>:"WPI_RobotDriveTankDrive.vi"("Right axis value"=1.0 ("Left axis value"), "Left axis value"=1.0 ("Right axis value"), "RobotDriveDevRef"=w1038) -> ()  [unwired: 6 in, 3 out]
                n457 = Greater?(x=w1037, y=u32 170) -> (0:w1035:bool)
                n458 = case shown="False" w1035 {
                  tunnel: [T4."ação 1" T4."ação 2"] -> w1034
                  frame False {
                  }
                  frame True {
                  }
                }
              }
            }
          }
          frame "ação 2" {
            n459 = call <vilib>:"WPI_RobotDriveTankDrive.vi"("Right axis value"=0.0, "Left axis value"=0.0, "RobotDriveDevRef"=w1043) -> ()  [unwired: 6 in, 3 out]
          }
          frame "ação 3" {
            n460 = local read "Sensor Position 4"() -> (w1056:dbl)
            n461 = call <vilib>:"Spark MAX Set Sensor Position.vi"("Position"=0.0, "MotorControlDeviceRef"=w1049) -> ()  [unwired: 8 in, 2 out]
            n462 = call <vilib>:"Spark MAX Set Sensor Position.vi"("Position"=0.0, "MotorControlDeviceRef"=w1048) -> ()  [unwired: 8 in, 2 out]
            n463 = Greater?(x=w1056, y=57.0) -> (0:w1057:bool)
            n464 = call <vilib>:"WPI_RobotDriveTankDrive.vi"("Right axis value"=0.5 ("Left axis value"), "Left axis value"=0.5, "RobotDriveDevRef"=w1060) -> ()  [unwired: 6 in, 3 out]
            n465 = case shown="False" w1057 {
              tunnel: w1054 -> [_ w1064]
              tunnel: [T4."ação 3" T4."ação 4"] -> w1052
              frame False {
              }
              frame True {
                n466 = call <vilib>:"Spark MAX Set Sensor Position.vi"("Position"=0.0, "MotorControlDeviceRef"=w1064) -> ()  [unwired: 8 in, 2 out]
              }
            }
          }
          frame "ação 4" {
            n467 = local read "Sensor Position 4"() -> (w1074:dbl)
            n468 = call <vilib>:"Spark MAX Set Sensor Position.vi"("Position"=0.0, "MotorControlDeviceRef"=w1065) -> ()  [unwired: 8 in, 2 out]
            n469 = call <vilib>:"Spark MAX Set Sensor Position.vi"("Position"=0.0, "MotorControlDeviceRef"=w1066) -> ()  [unwired: 8 in, 2 out]
            n470 = call <vilib>:"WPI_RobotDriveTankDrive.vi"("Right axis value"=-0.5 ("Left axis value"), "Left axis value"=0.5, "RobotDriveDevRef"=w1077) -> ()  [unwired: 6 in, 3 out]
            n471 = Greater?(x=w1074, y=14.0) -> (0:w1072:bool)
            n472 = case shown="True" w1072 {
              tunnel: w1071 -> [_ w1081]
              tunnel: [T4."ação 4" T4."ação 5"] -> w1069
              frame False {
              }
              frame True {
                n473 = call <vilib>:"Spark MAX Set Sensor Position.vi"("Position"=0.0, "MotorControlDeviceRef"=w1081) -> ()  [unwired: 8 in, 2 out]
              }
            }
          }
          frame "ação 5" {
            n474 = local read "Sensor Position 4"() -> (w1090:dbl)
            n475 = call <vilib>:"Spark MAX Set Sensor Position.vi"("Position"=0.0, "MotorControlDeviceRef"=w1083) -> ()  [unwired: 8 in, 2 out]
            n476 = call <vilib>:"WPI_RobotDriveTankDrive.vi"("Right axis value"=-0.5 ("Left axis value"), "Left axis value"=-0.5, "RobotDriveDevRef"=w1091) -> ("RobotDriveDevRef"=w1088:T5)  [unwired: 6 in, 2 out]
            n477 = call <vilib>:"Spark MAX Set Sensor Position.vi"("Position"=0.0, "MotorControlDeviceRef"=w1082) -> ()  [unwired: 8 in, 2 out]
            n478 = Less?(x=w1090, y=-50.0) -> (x < y?=w1086:bool)
            n479 = case shown="True" w1086 {
              tunnel: w1088 -> [_ w1094]
              frame False {
              }
              frame True {
                n480 = call <vilib>:"WPI_RobotDriveTankDrive.vi"("Right axis value"=0.0 ("Left axis value"), "Left axis value"=0.0, "RobotDriveDevRef"=w1094) -> ()  [unwired: 6 in, 3 out]
              }
            }
          }
        }
      }
    }
    frame "teste shooter" {
      n481 = call <vilib>:"WPI_RobotDriveRefNum Registry Get.vi"("refnum name"="rd") -> ("RobotDriveDevRef"=w1102:T5)  [unwired: 9 in, 1 out]
      n482 = call <vilib>:"WPI_RobotDriveTankDrive.vi"("Right axis value"=1.0 ("Left axis value"), "Left axis value"=1.0, "RobotDriveDevRef"=w1102) -> ("RobotDriveDevRef"=w1097:T5)  [unwired: 6 in, 2 out]
      n483 = Unbundle By Name(w1097) -> ("Motors[]"=w1098:T6[])
      n484 = while {
        tunnel: w1098 -> [w1110]
        stop <- w1107 stop-if-true
        n485 = Index Array(array=w1110) -> (element #1=w1115:T6, element #2=w1114:T6)  [unwired: 2 in]
        n486 = Wait (ms)(milliseconds to wait=u32 20) -> ()  [unwired: 1 out]
        n487 = call <vilib>:"Spark MAX Get Sensor Position.vi"("MotorControlDevRef in"=w1114) -> ("Sensor Position"=w1113:dbl, "MotorControlDevRef out"=w1105:T6)  [unwired: 7 in, 2 out]
        "Sensor Position 7" <- w1113
        n488 = call <vilib>:"Spark MAX Get Sensor Position.vi"("MotorControlDevRef in"=w1115) -> ("Sensor Position"=w1103:dbl, "MotorControlDevRef out"=w1104:T6)  [unwired: 7 in, 2 out]
        "Sensor Position 8" <- w1103
        n489 = Greater?(x=w1113, y=50.0) -> (0:w1108:bool)
        n490 = Greater?(x=w1103, y=50.0) -> (0:w1109:bool)
        n491 = And(x=w1109, y=w1108) -> (x .and. y?=w1107:bool)
        n492 = case shown="True" w1109 {
          tunnel: w1104 -> [_ w1123]
          frame False {
          }
          frame True {
            n493 = call <vilib>:"WPI_MotorControlSetOutput.vi"("Output"=0.0, "MotorControlDevRef"=w1123) -> ("MotorControlDevRef"=w1121:T6)  [unwired: 7 in, 2 out]
            n494 = call <vilib>:"Spark MAX Set Sensor Position.vi"("Position"=0.0, "MotorControlDeviceRef"=w1121) -> ()  [unwired: 8 in, 2 out]
          }
        }
        n495 = case shown="True" w1108 {
          tunnel: w1105 -> [_ w1119]
          frame False {
          }
          frame True {
            n496 = call <vilib>:"WPI_MotorControlSetOutput.vi"("Output"=0.0, "MotorControlDevRef"=w1119) -> ("MotorControlDevRef"=w1117:T6)  [unwired: 7 in, 2 out]
            n497 = call <vilib>:"Spark MAX Set Sensor Position.vi"("Position"=0.0, "MotorControlDeviceRef"=w1117) -> ()  [unwired: 8 in, 2 out]
          }
        }
      }
    }
  }
